vi "LeakageFenxi.vi"(7 "采样时间":string, 8 "Area_name":string, 9 "采样数据":string[][](array[string]), 10 "是否存在记录":bool=TRUE, 11 "3DData":cluster{"X":dbl[], "Y":dbl[], "Z":dbl[]}) -> ()   [LabVIEW 2014, in "cyy.lvlib" / "LeakageFenXi.lvlib"]
uses:
  LeakageFenXi.lvlib
  <vilib>/Math Plots/3D Math Plots/3D Contour/3D Contour XCtrl/3D Contour.xctl
  <vilib>/Math Plots/3D Math Plots/3D Surface/3D Surface XCtrl/3D Surface.xctl
  <vilib>/Math Plots/3D Math Plots/3D Mesh/3D Mesh XCtrl/3D Mesh.xctl
  <vilib>/imath/engines/lvmath2/RunTimeEngine/Managers/WorkSpace/UID Generator.vi
  <vilib>/imath/engines/lvmath2/RunTimeEngine/RunTimeType/NIMS_RunTimeType_From StrictType (excl LVString).vi
  <instcachedir>/0/NIMS_RunTimeType_From StrictType (excl LVString)_15A5391EEA9C4AACB9955AC755B83D29.lvgen/NIMS_RunTimeType_From StrictType (excl LVString)_15A5391EEA9C4AACB9955AC755B83D29_000.vi
  <vilib>/imath/engines/lvmath2/RunTimeEngine/LocalVariableDefStatement/MC_LocalVariableDefStatement_Display.vi
  <vilib>/imath/engines/lvmath2/RunTimeEngine/BuiltInFunctions/max/1 input/NIMS_max(RV).vi
  <instcachedir>/0/NIMS_max(RV)_237633DB1D604D5BA7001287DF3C7957.lvgen/NIMS_max(RV)_237633DB1D604D5BA7001287DF3C7957_000.vi
  <vilib>/imath/engines/lvmath2/RunTimeEngine/BuiltInFunctions/min/1 input/NIMS_min(RV).vi
  <instcachedir>/0/NIMS_min(RV)_EE2DD3E2888846108C5160A664B67832.lvgen/NIMS_min(RV)_EE2DD3E2888846108C5160A664B67832_000.vi
  <vilib>/imath/engines/lvmath2/RunTimeEngine/BuiltInFunctions/linramp/NIMS_linramp.vi
  <vilib>/imath/engines/lvmath2/RunTimeEngine/BuiltInFunctions/meshgrid2d/NIMS_meshgrid2d(V,V).vi
  <instcachedir>/0/NIMS_meshgrid2d(V,V)_3733343E1C554A708015CFB0432C6A59.lvgen/NIMS_meshgrid2d(V,V)_3733343E1C554A708015CFB0432C6A59_000.vi
  <vilib>/imath/engines/lvmath2/RunTimeEngine/BuiltInFunctions/intrp2d_uneven/NIMS_[1o]_intrp2d_uneven.vi
  <vilib>/imath/engines/lvmath2/RunTimeEngine/ErrorHandling/NIMS_Error From Error Code.vi
  <vilib>/imath/engines/lvmath2/RunTimeEngine/VariableToken/NIMS_VariableToken_CondDefined.vi
  <instcachedir>/0/NIMS_VariableToken_CondDefined_EE8DD211A89249938CE6537267F5C9B3.lvgen/NIMS_VariableToken_CondDefined_EE8DD211A89249938CE6537267F5C9B3_001.vi
  <vilib>/imathl/engines/lvmath/Functions/Error Handling/Create Error.vi
  <vilib>/imath/engines/lvmath/Functions/Error Handling/MergeErrorsWrapper.vi
  <vilib>/imath/engines/lvmath2/RunTimeEngine/Managers/SymbolTable/Clear UID.vi
  <vilib>/imath/engines/lvmath2/RunTimeEngine/NodeEndStatement/NIMS_NodeEndStatement_Output.vi
  <instcachedir>/0/NIMS_NodeEndStatement_Output_53EC0D466D134D7ABD903AC30B43404B.lvgen/NIMS_NodeEndStatement_Output_53EC0D466D134D7ABD903AC30B43404B_012.vi
  <instcachedir>/0/NIMS_NodeEndStatement_Output_53EC0D466D134D7ABD903AC30B43404B.lvgen/NIMS_NodeEndStatement_Output_53EC0D466D134D7ABD903AC30B43404B_002.vi
  <vilib>/imath/engines/lvmath2/RunTimeEngine/ErrorHandling/NIMS_Finalize Error.vi
  <vilib>/Utility/file.llb/Write To Spreadsheet File (string).vi
  <vilib>/imath/engines/lvmath2/RunTimeEngine/RangeToken/NIMS_Range_R2 - Integer.vi
  <instcachedir>/0/NIMS_Range_R2 - Integer_2D1304BAF97744E0A293025746CBADFC.lvgen/NIMS_Range_R2 - Integer_2D1304BAF97744E0A293025746CBADFC_000.vi
  <vilib>/imath/engines/lvmath2/RunTimeEngine/CommandStatement/MC_CommandStatement_break.vi
  <vilib>/imath/engines/lvmath2/RunTimeEngine/IndexRead/NIMS V(S).vi
  <instcachedir>/0/NIMS V(S)_0488751826AF41519A22953C041130DC.lvgen/NIMS V(S)_0488751826AF41519A22953C041130DC_000.vi
  <vilib>/imath/engines/lvmath2/RunTimeEngine/ArithmeticOperatorToken/NIMS_ArithmeticOperator_times.vi
  <instcachedir>/0/NIMS_ArithmeticOperator_times_2EFF5B13FCA4492A81D59089AD809F54.lvgen/NIMS_ArithmeticOperator_times_2EFF5B13FCA4492A81D59089AD809F54_007.vi
  <vilib>/imath/engines/lvmath2/RunTimeEngine/ArithmeticOperatorToken/NIMS_ArithmeticOperator_plus.vi
  <instcachedir>/0/NIMS_ArithmeticOperator_plus_48D6EAACA5D645B09F7EC9C016C2DEA8.lvgen/NIMS_ArithmeticOperator_plus_48D6EAACA5D645B09F7EC9C016C2DEA8_003.vi
  <vilib>/imath/engines/lvmath2/RunTimeEngine/ErrorHandling/NIMS_Create Error From Enums.vi
  <instcachedir>/0/NIMS_ArithmeticOperator_plus_48D6EAACA5D645B09F7EC9C016C2DEA8.lvgen/NIMS_ArithmeticOperator_plus_48D6EAACA5D645B09F7EC9C016C2DEA8_002.vi
  <vilib>/imath/engines/lvmath2/RunTimeEngine/BuiltInFunctions/abs/NIMS_abs(signed).vi
  <instcachedir>/0/NIMS_abs(signed)_C4FCB8E6058B49B797C7C8D53CA5F6EC.lvgen/NIMS_abs(signed)_C4FCB8E6058B49B797C7C8D53CA5F6EC_000.vi
  <instcachedir>/0/NIMS_ArithmeticOperator_times_2EFF5B13FCA4492A81D59089AD809F54.lvgen/NIMS_ArithmeticOperator_times_2EFF5B13FCA4492A81D59089AD809F54_001.vi
  <vilib>/imath/engines/lvmath2/RunTimeEngine/IndexReplace/NIMS M($,$)=M.vi
  <instcachedir>/0/NIMS M($,$)=M_01E89DEB123E4D8BA4D741A9F51B9E5E.lvgen/NIMS M($,$)=M_01E89DEB123E4D8BA4D741A9F51B9E5E_002.vi
  <vilib>/imath/engines/lvmath2/RunTimeEngine/IndexReplace/NIMS M(S,S)=S.vi
  <instcachedir>/0/NIMS M(S,S)=S_43446D47E75543269C90719353EB0EB0.lvgen/NIMS M(S,S)=S_43446D47E75543269C90719353EB0EB0_001.vi
  <vilib>/imath/engines/lvmath2/RunTimeEngine/IndexRead/NIMS M($,$).vi
  <instcachedir>/0/NIMS M($,$)_A19103A80C29478F88F4B4F0744DBFE6.lvgen/NIMS M($,$)_A19103A80C29478F88F4B4F0744DBFE6_000.vi
  <vilib>/imath/engines/lvmath2/RunTimeEngine/BuiltInFunctions/max/1 input/NIMS_max(CM).vi
  <instcachedir>/0/NIMS_max(CM)_07A280EFFE444116B5339E96F9201E32.lvgen/NIMS_max(CM)_07A280EFFE444116B5339E96F9201E32_000.vi
  <vilib>/imath/engines/lvmath2/RunTimeEngine/BuiltInFunctions/min/1 input/NIMS_min(CV).vi
  <instcachedir>/0/NIMS_min(CV)_813D140E220645C2A7BAD197162D0D3E.lvgen/NIMS_min(CV)_813D140E220645C2A7BAD197162D0D3E_000.vi
  <instcachedir>/0/NIMS V(S)_0488751826AF41519A22953C041130DC.lvgen/NIMS V(S)_0488751826AF41519A22953C041130DC_002.vi
  <instcachedir>/0/NIMS_NodeEndStatement_Output_53EC0D466D134D7ABD903AC30B43404B.lvgen/NIMS_NodeEndStatement_Output_53EC0D466D134D7ABD903AC30B43404B_005.vi
  <vilib>/Math Plots/3D Math Plots/3D Contour/3D Contour Datatype/Public/Plot Helper (Matrix).vi
  <vilib>/imath/engines/lvmath2/RunTimeEngine/BuiltInFunctions/max/1 input/NIMS_max(RM).vi
  <instcachedir>/0/NIMS_max(RM)_8387F852894F4122B05F4338BED9FDFF.lvgen/NIMS_max(RM)_8387F852894F4122B05F4338BED9FDFF_000.vi
  <vilib>/Math Plots/3D Math Plots/3D Surface/3D Surface Datatype/Public/Plot Helper (Matrix).vi
  <vilib>/Math Plots/3D Math Plots/3D Mesh/3D Mesh Datatype/Public/Plot Helper (Matrix).vi
  <vilib>/Math Plots/3D Math Plots/3D Contour/3D Contour Datatype/3D Contour Datatype.lvclass
  <vilib>/imath/engines/lvmath2/RunTimeEngine/Managers/SymbolTable/NIMS_WorkSpace.lvlib
  <vilib>/Math Plots/3D Math Plots/3D Surface/3D Surface Datatype/3D Surface Datatype.lvclass
  <vilib>/Math Plots/3D Math Plots/3D Mesh/3D Mesh Datatype/3D Mesh Datatype.lvclass
  CYY/cyy.lvlib
  DataBase/DataBase.lvlib
panel:
  in  "预警":bool
  in  "查看采样数据":bool
  out "当前采样分析信息":string
  out "最大索引":u32[](array[numeric])
  out "数字":dbl[](array[numeric]) format="%#.6g"
  out "数字 2":dbl[](array[numeric]) format="%#.6g"
  in  "退出":bool
  in  "分析":bool
  in  "预判":bool
  in  "预判方式":u16(ring) items=["linear", "cubic", "nearest"]
  in  "导出数据":bool
  in  "三维网格图":bool
  in  "三维曲面图":bool
  in  "三维等高线":bool
  out "预判点":string
  out "渗漏点":string
  in  "MMM":bool
  in  "选项卡控件":enum32{"三维曲面图", "三维等高线图", "三维网格图", "采样数据"}(tab)
  out "3D Surface":refnum<class "3D Plot Datatype.lvclass">[](xcontrol) caption="三维曲面"
  out "3D等高线":refnum<class "3D Plot Datatype.lvclass">[](xcontrol) caption="三维等高线"
  out "3D Mesh":refnum<class "3D Plot Datatype.lvclass">[](xcontrol) caption="三维网格"
  in  "采样数据":i32(listbox)
  out "导出数据位置":path
  out "Z索引":i32
  out "Y坐标":dbl
  out "X坐标":dbl
  out "Zmax":dbl
  out "绘图坐标Y":dbl
  out "绘图坐标X":dbl
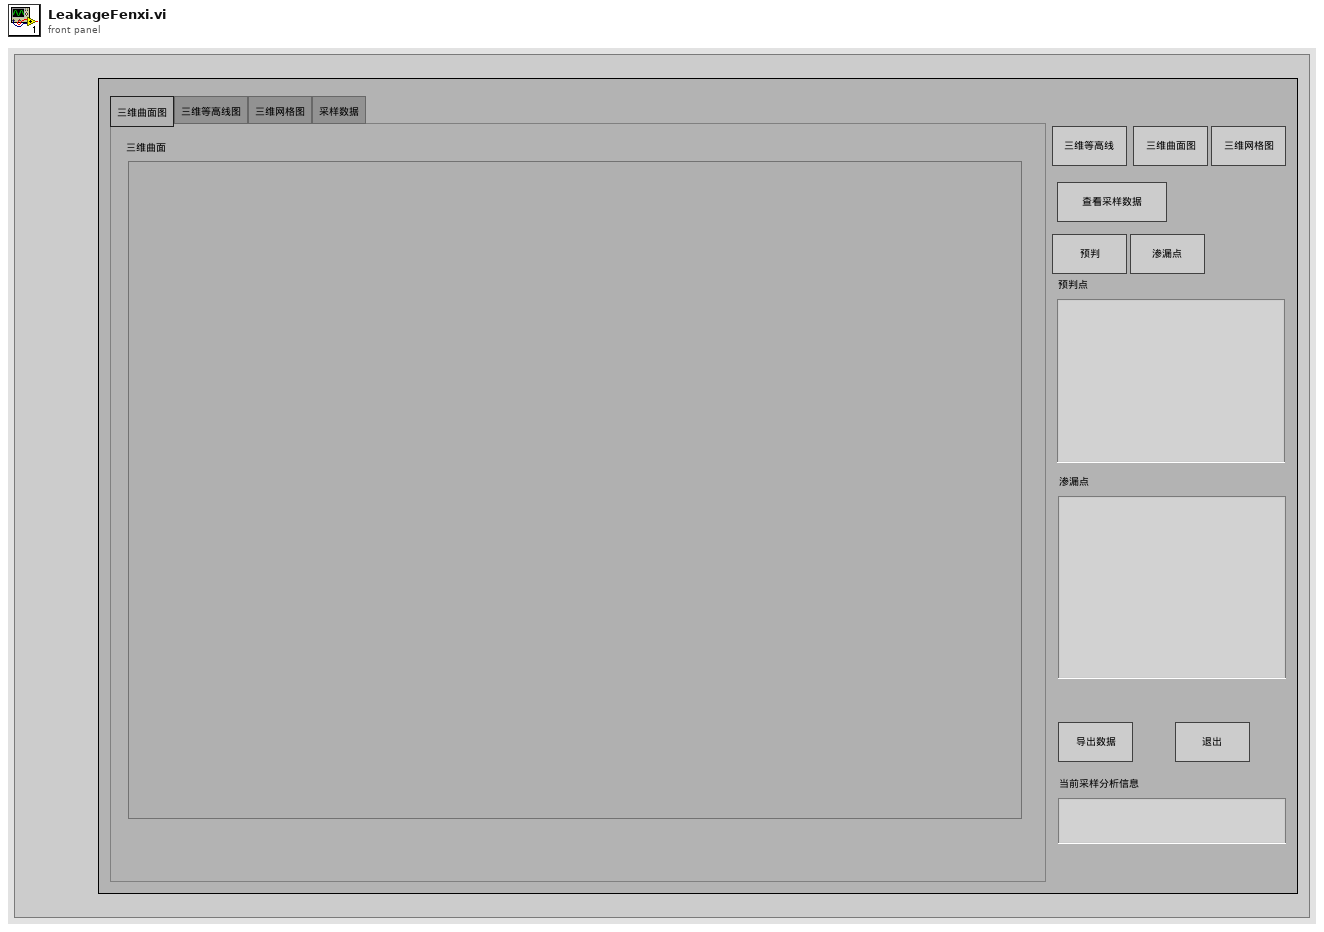
[diagram p1: front panel]
types:
  T1 = enum32{"invalid app kind", "Development System", "Run Time System", "Student Edition", "Embedded LabVIEW", "Evaluation", "Custom"}
  T2 = enum32{"Invalid", "Standard", "Closed", "Hidden", "Minimized", "Maximized"}
  T3 = cluster{"Core":cluster{"Current VI Reference":refnum<vi>, "Close Panel on Exit?":bool}, "Your Boolean data":bool, "Your string data":string, "3DData":cluster{"X":dbl[], "Y":dbl[], "Z":dbl[]}, "是否存在记录":bool, "采样数据":string[][], "SampleTime":string, "插值方式":i32, "Area_name":string, "坐标关系":cluster{"绘图坐标X":string, "绘图坐标Y":string, "实际坐标":string[]}, "是否进行预判":bool, "是否进行预警":bool}
  T4 = cluster{"绘图坐标X":string, "绘图坐标Y":string, "实际坐标":string[]}
  T5 = cluster{"Current VI Reference":refnum<vi>, "Close Panel on Exit?":bool}
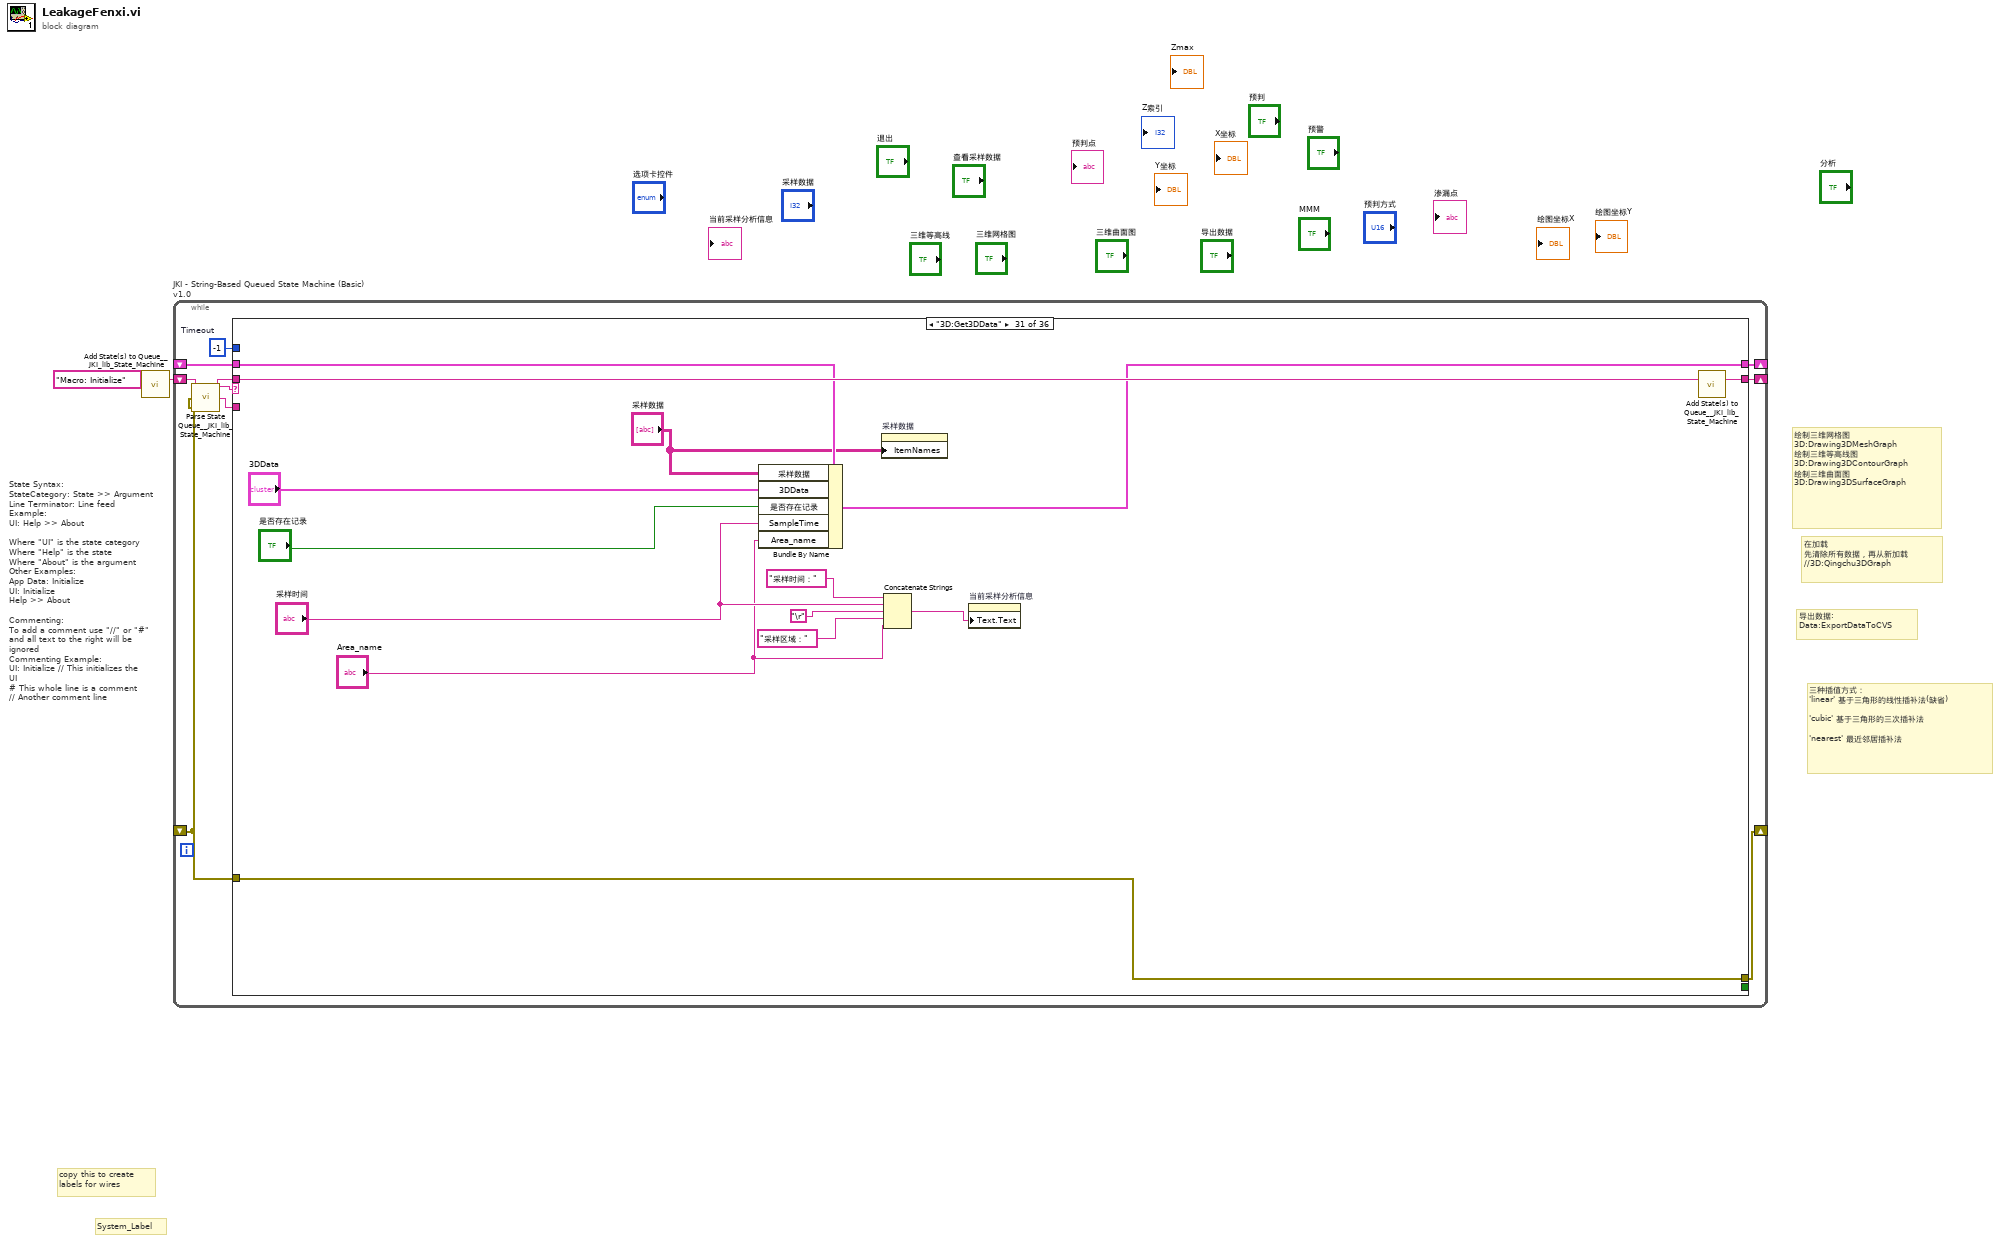
[diagram p0: block diagram]
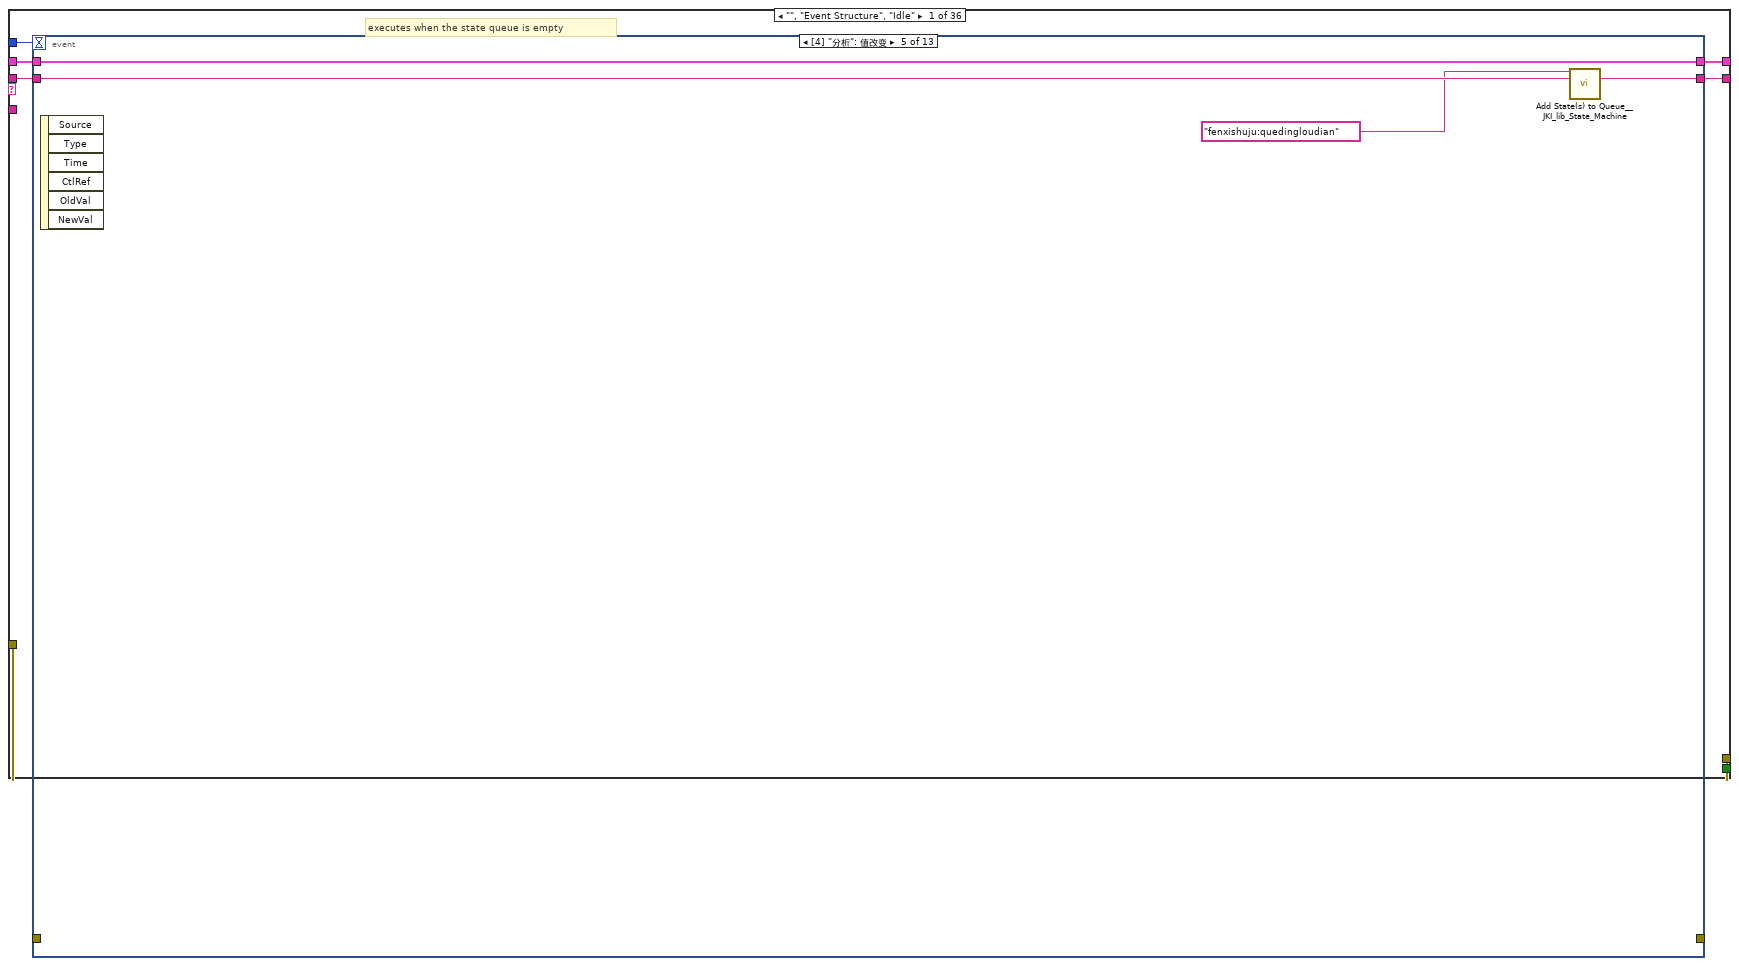
[diagram p2: hidden frame]
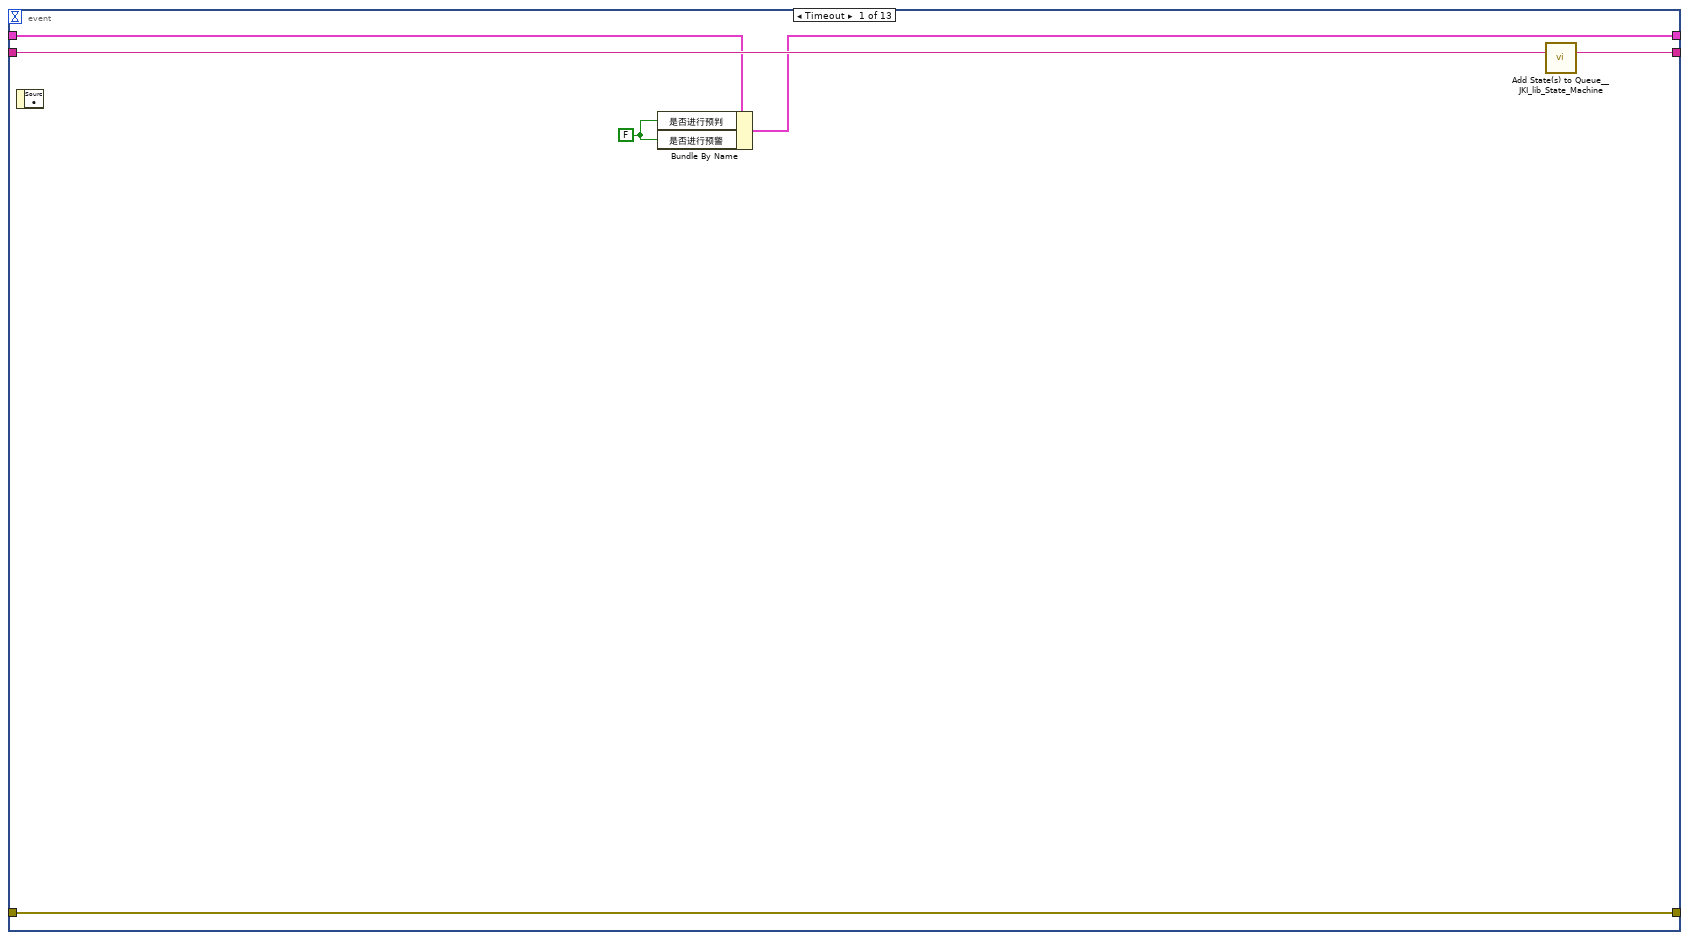
[diagram p3: hidden frame]
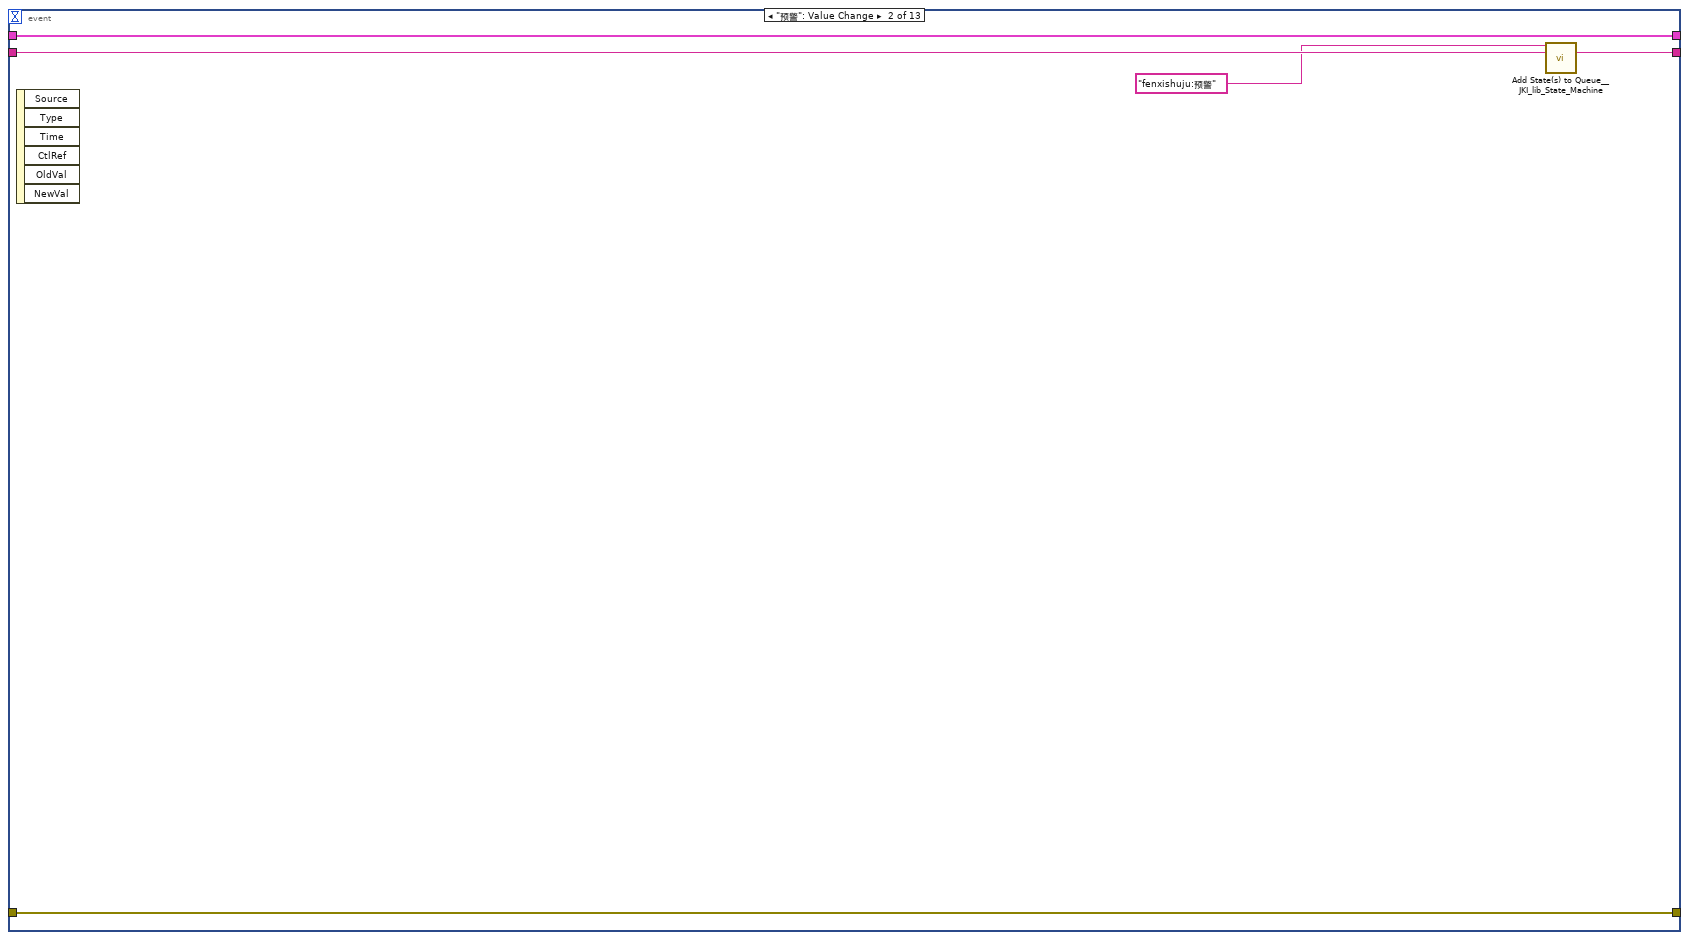
[diagram p4: hidden frame]
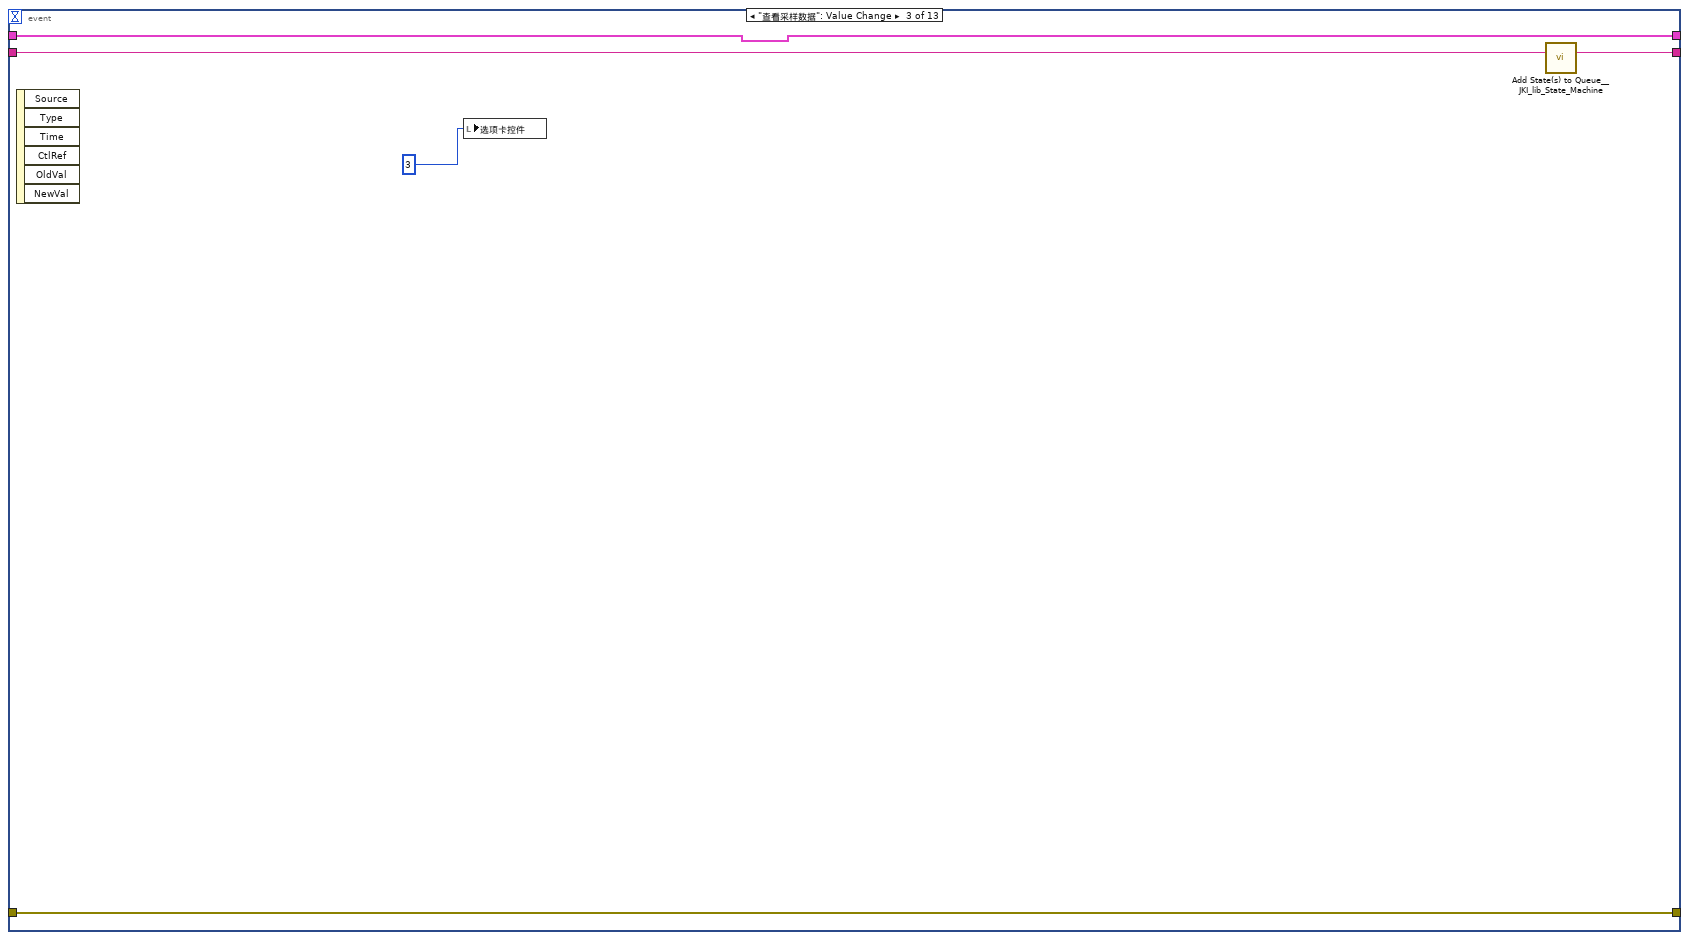
[diagram p5: hidden frame]
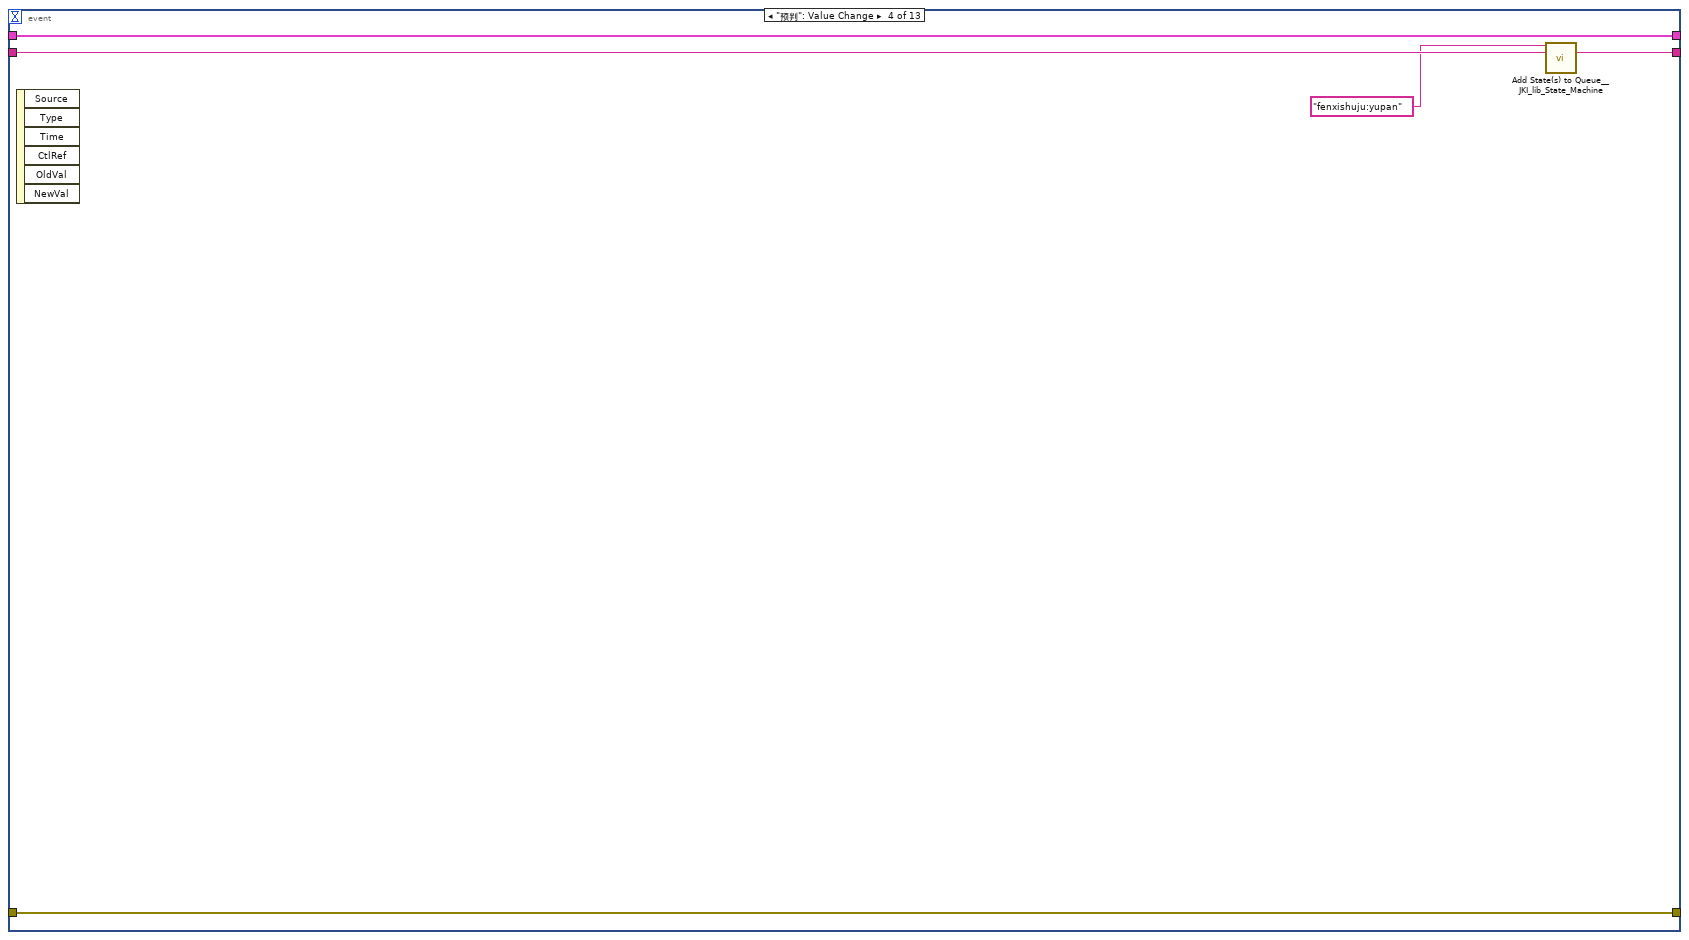
[diagram p6: hidden frame]
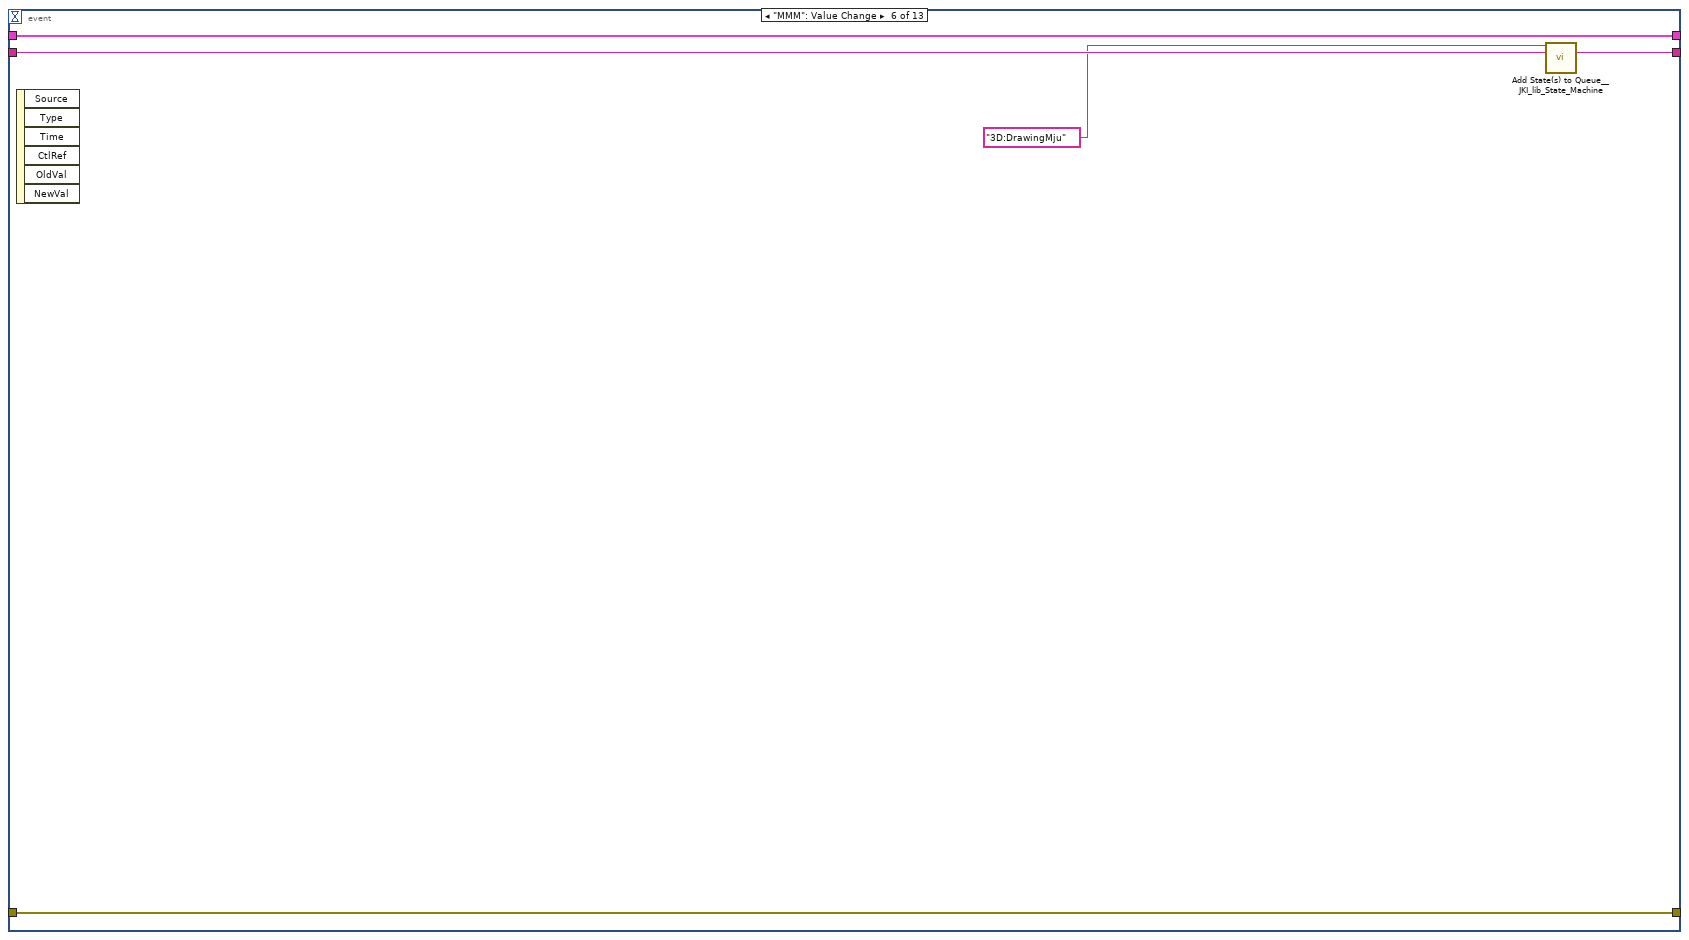
[diagram p7: hidden frame]
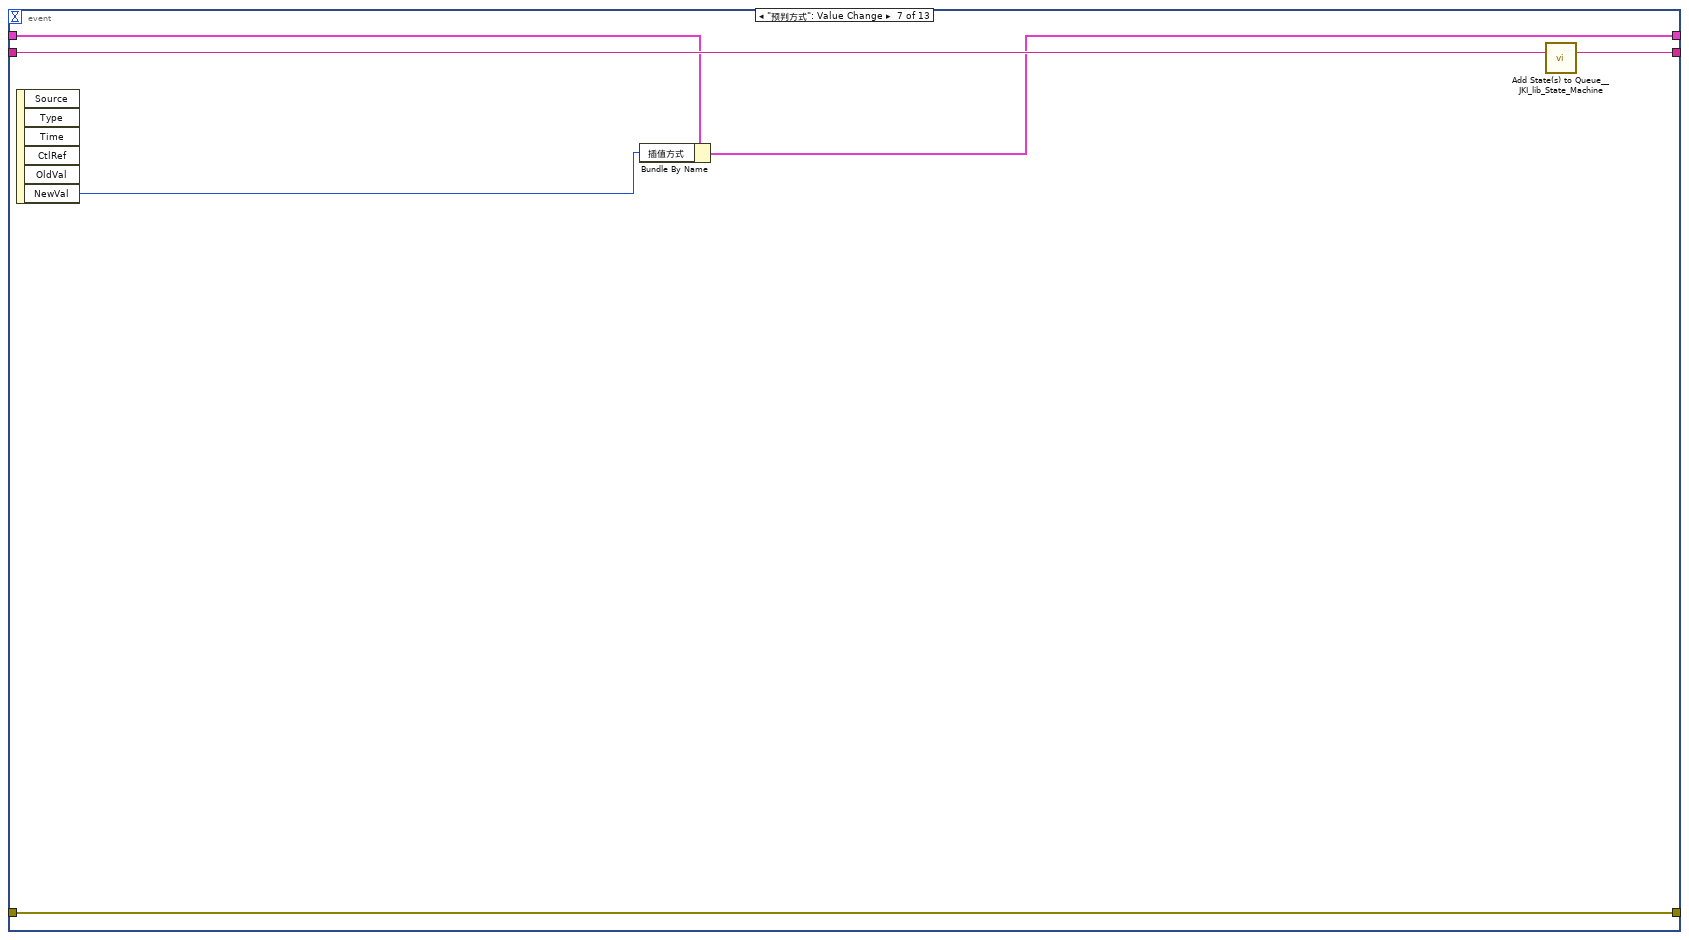
[diagram p8: hidden frame]
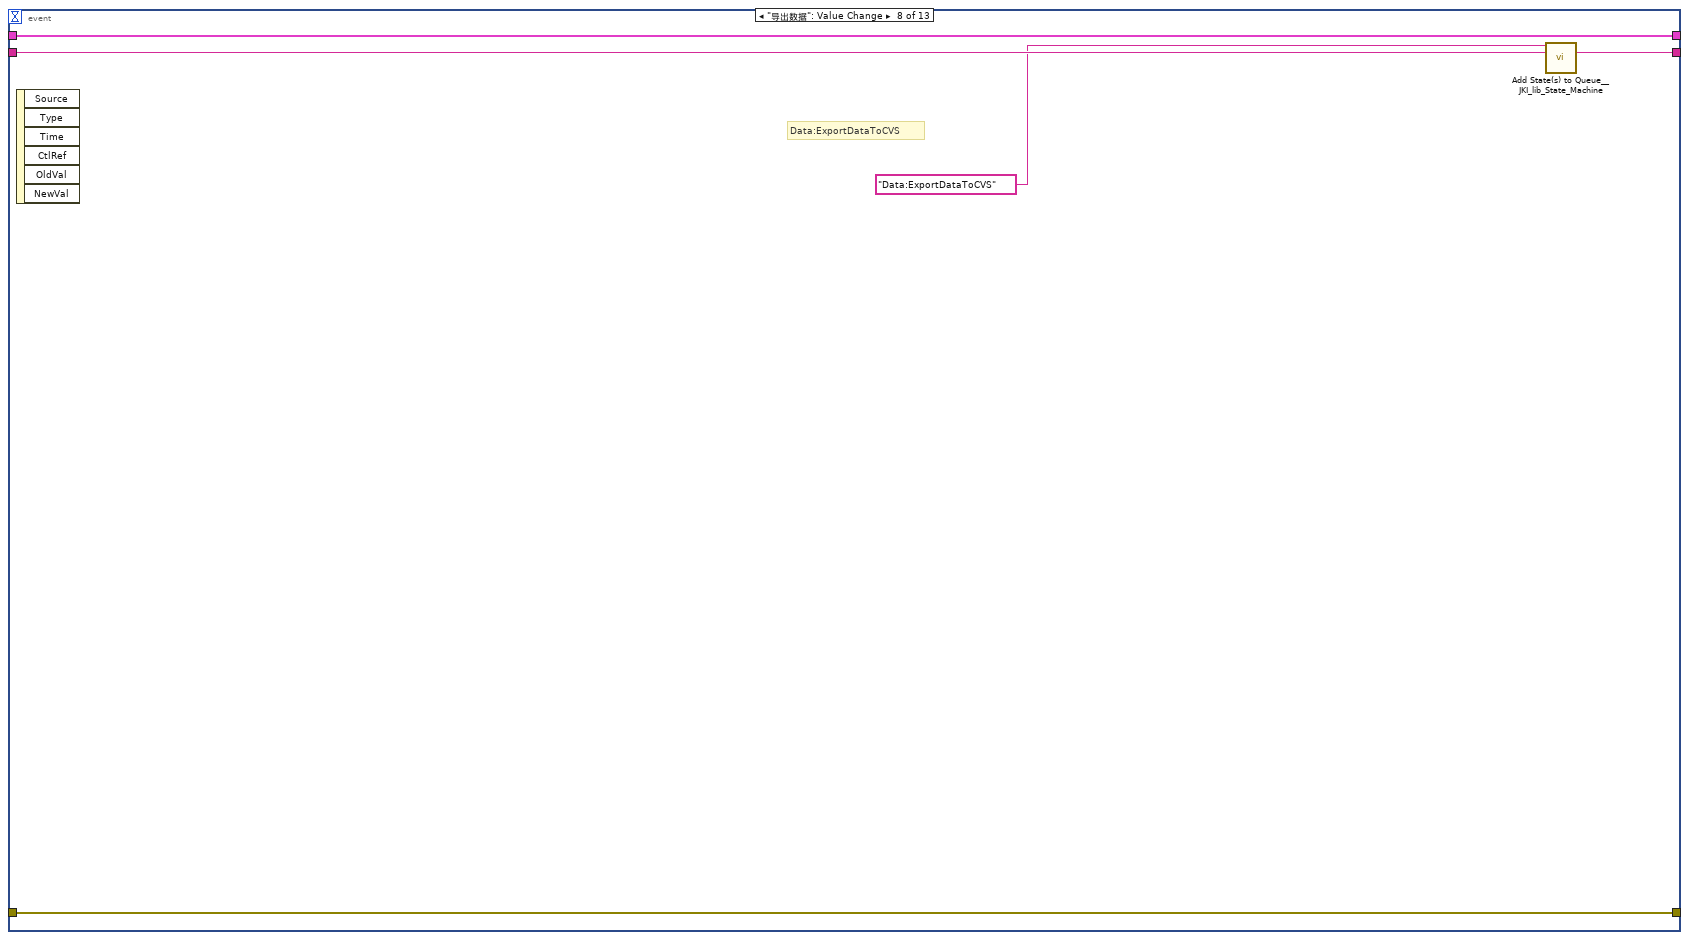
[diagram p9: hidden frame]
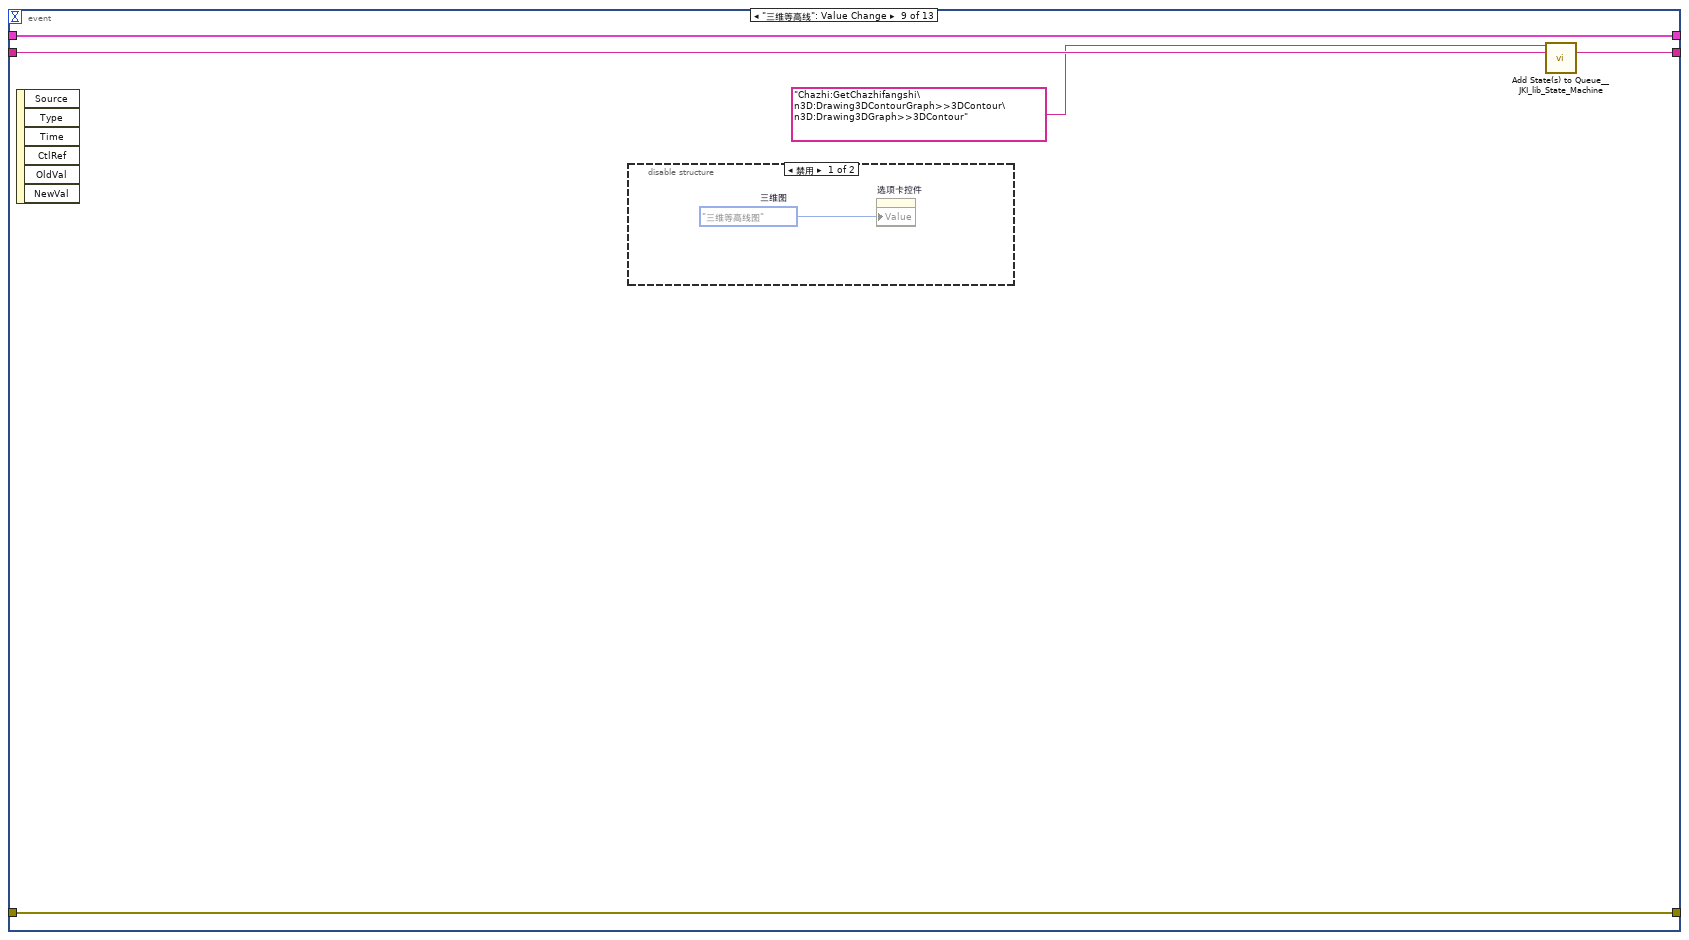
[diagram p10: hidden frame]
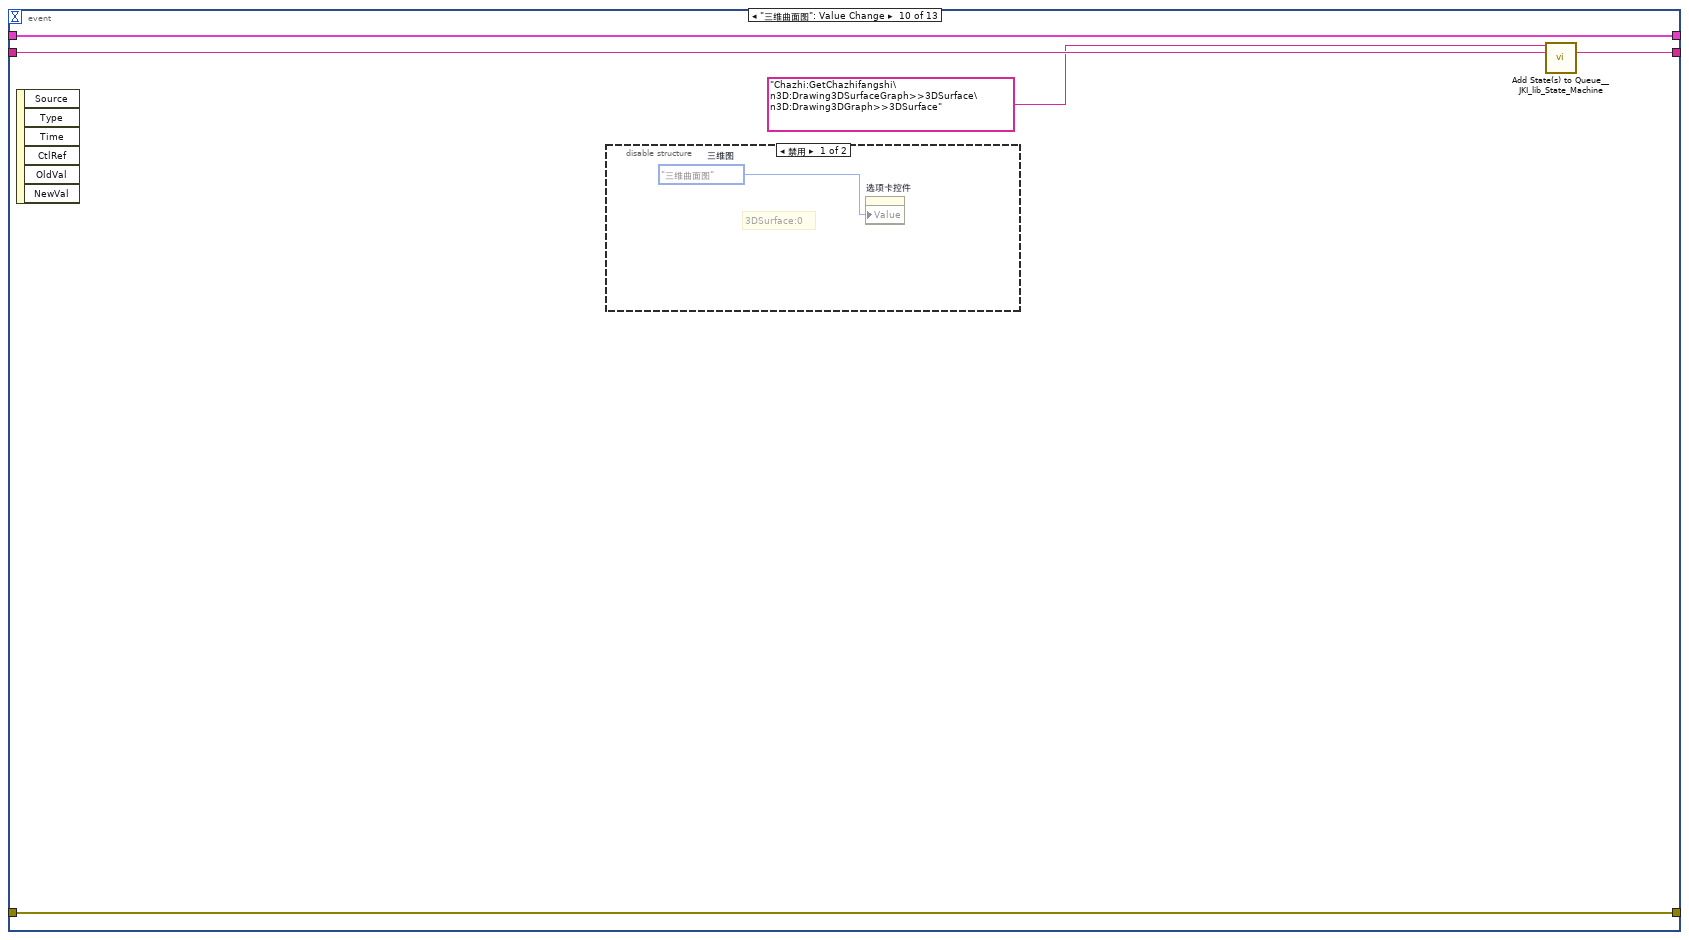
[diagram p12: hidden frame]
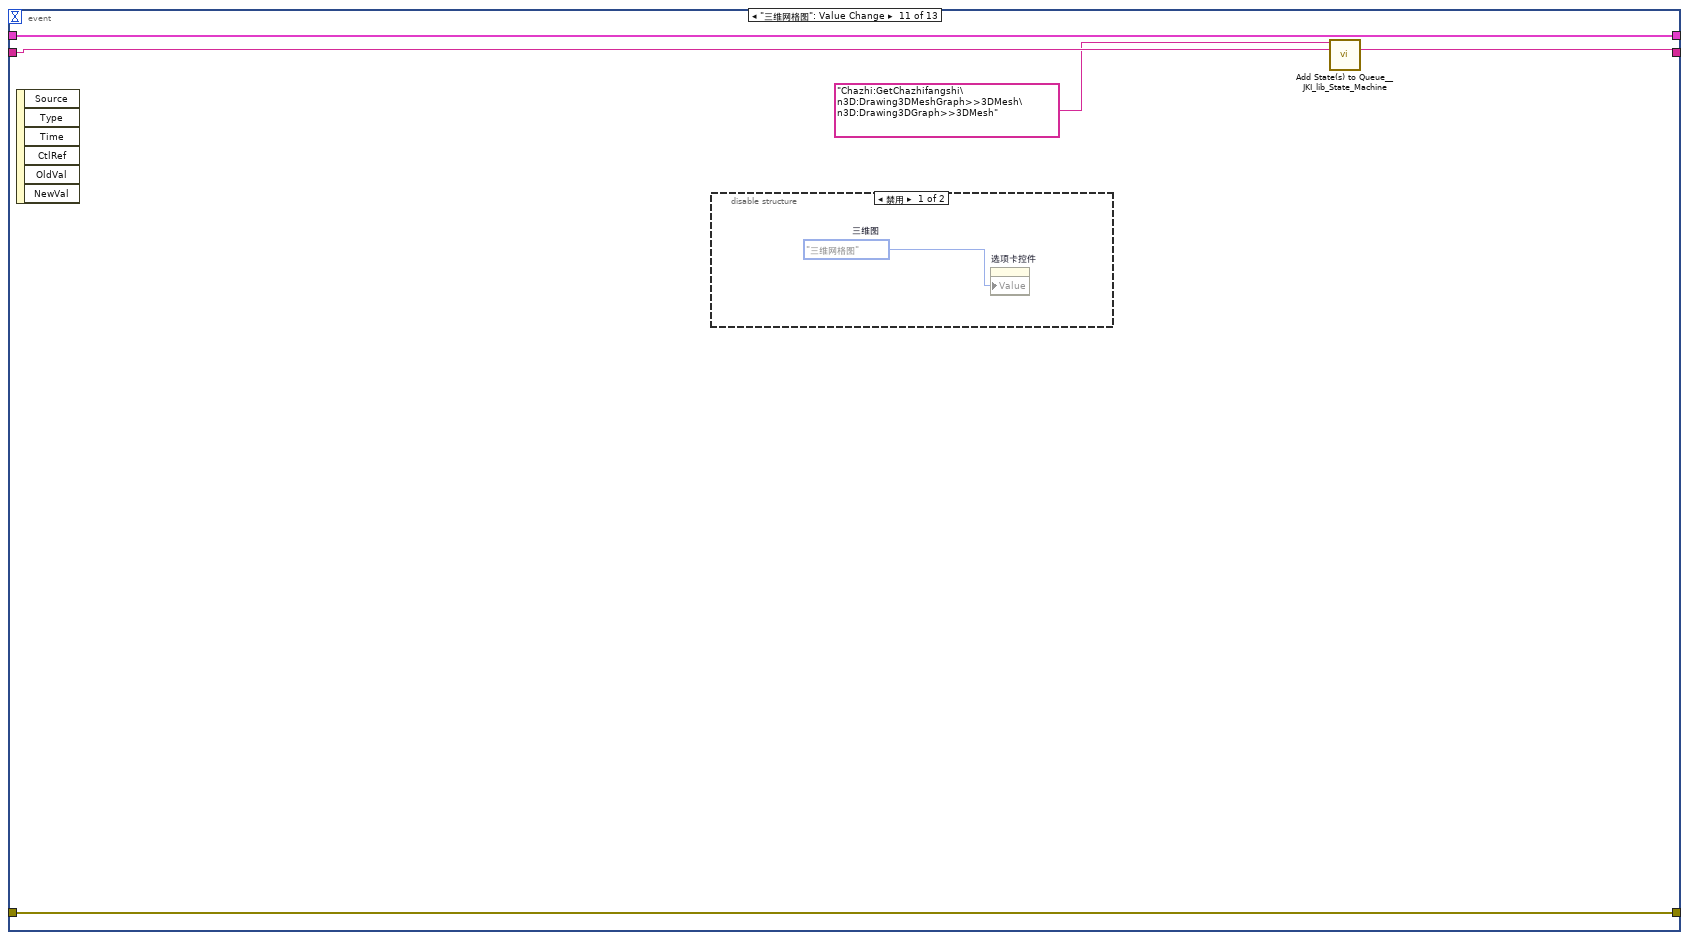
[diagram p14: hidden frame]
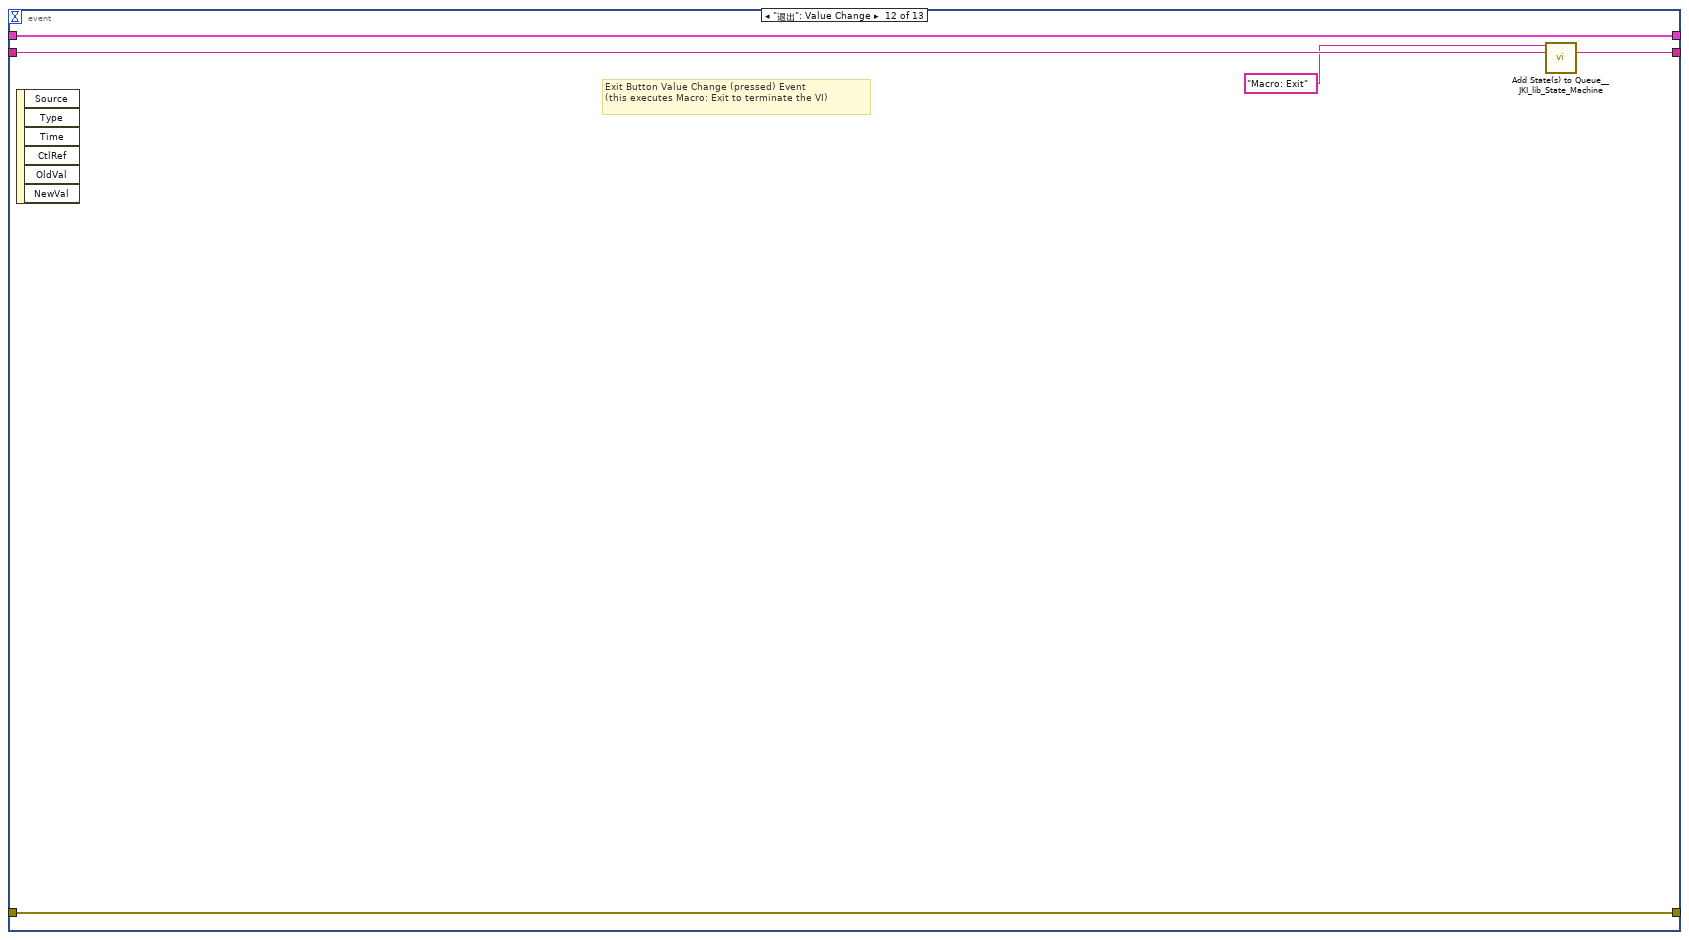
[diagram p16: hidden frame]
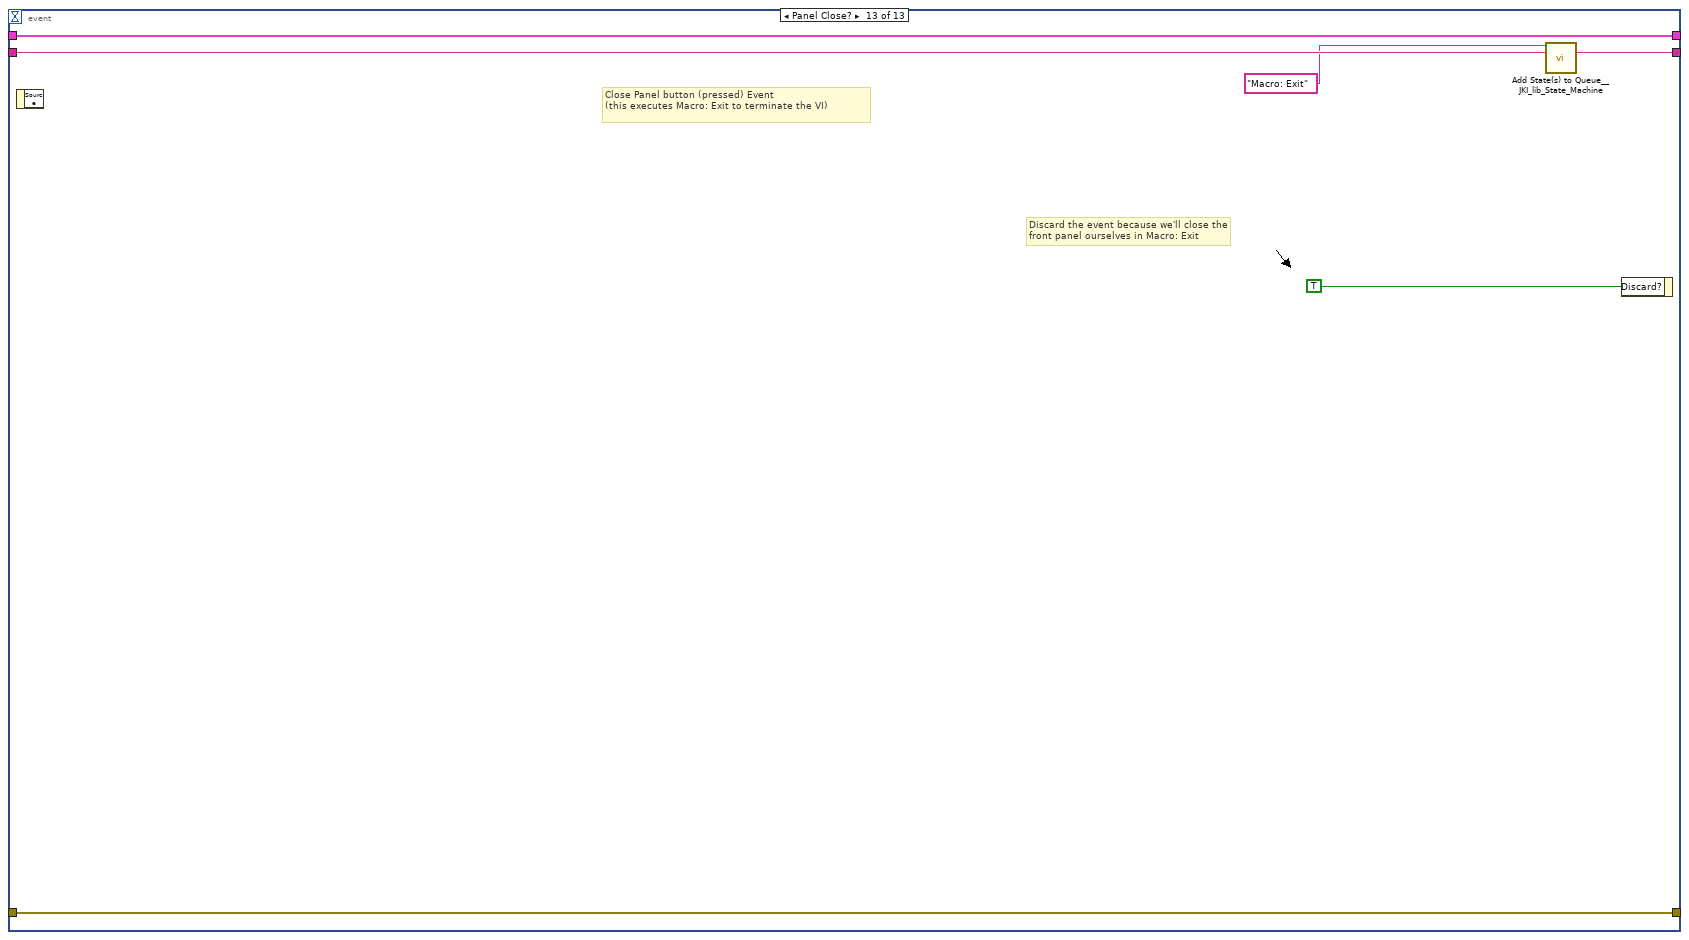
[diagram p17: hidden frame]
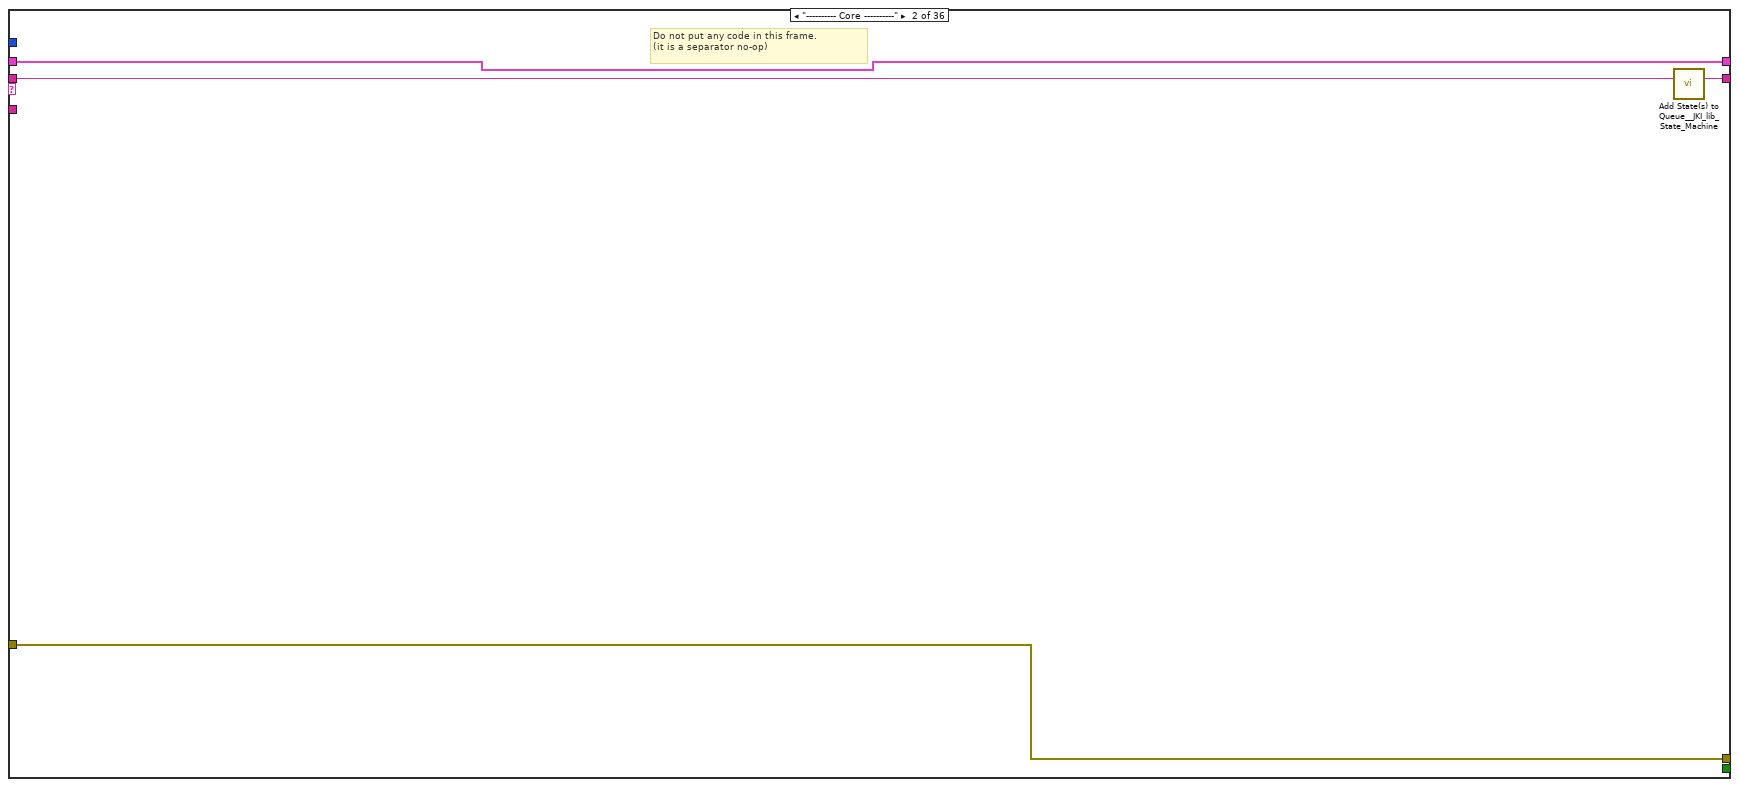
[diagram p18: hidden frame]
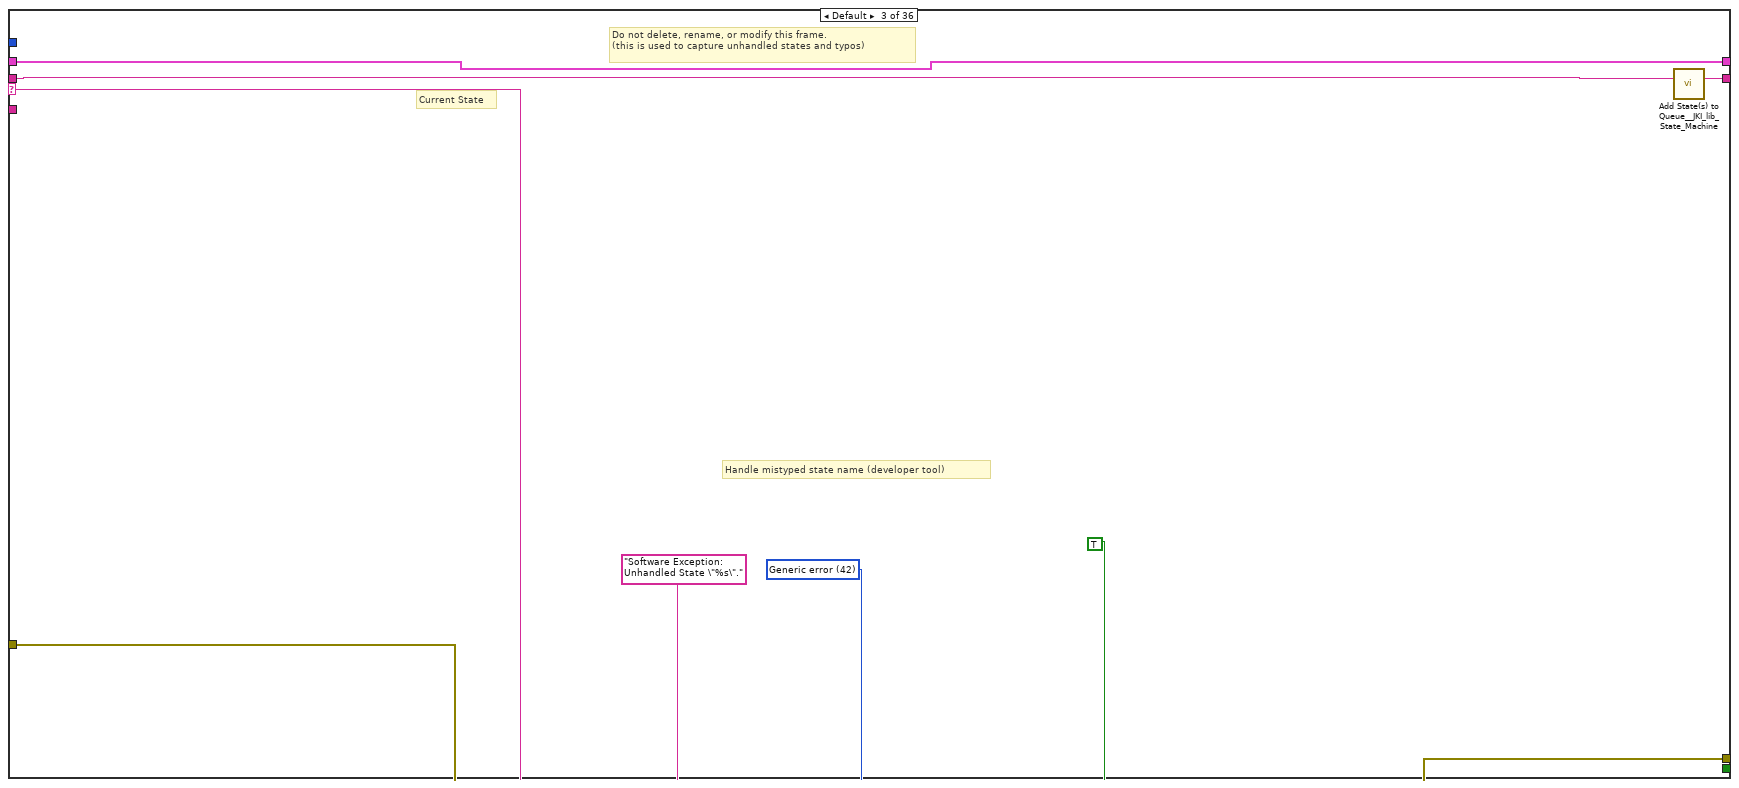
[diagram p19: hidden frame]
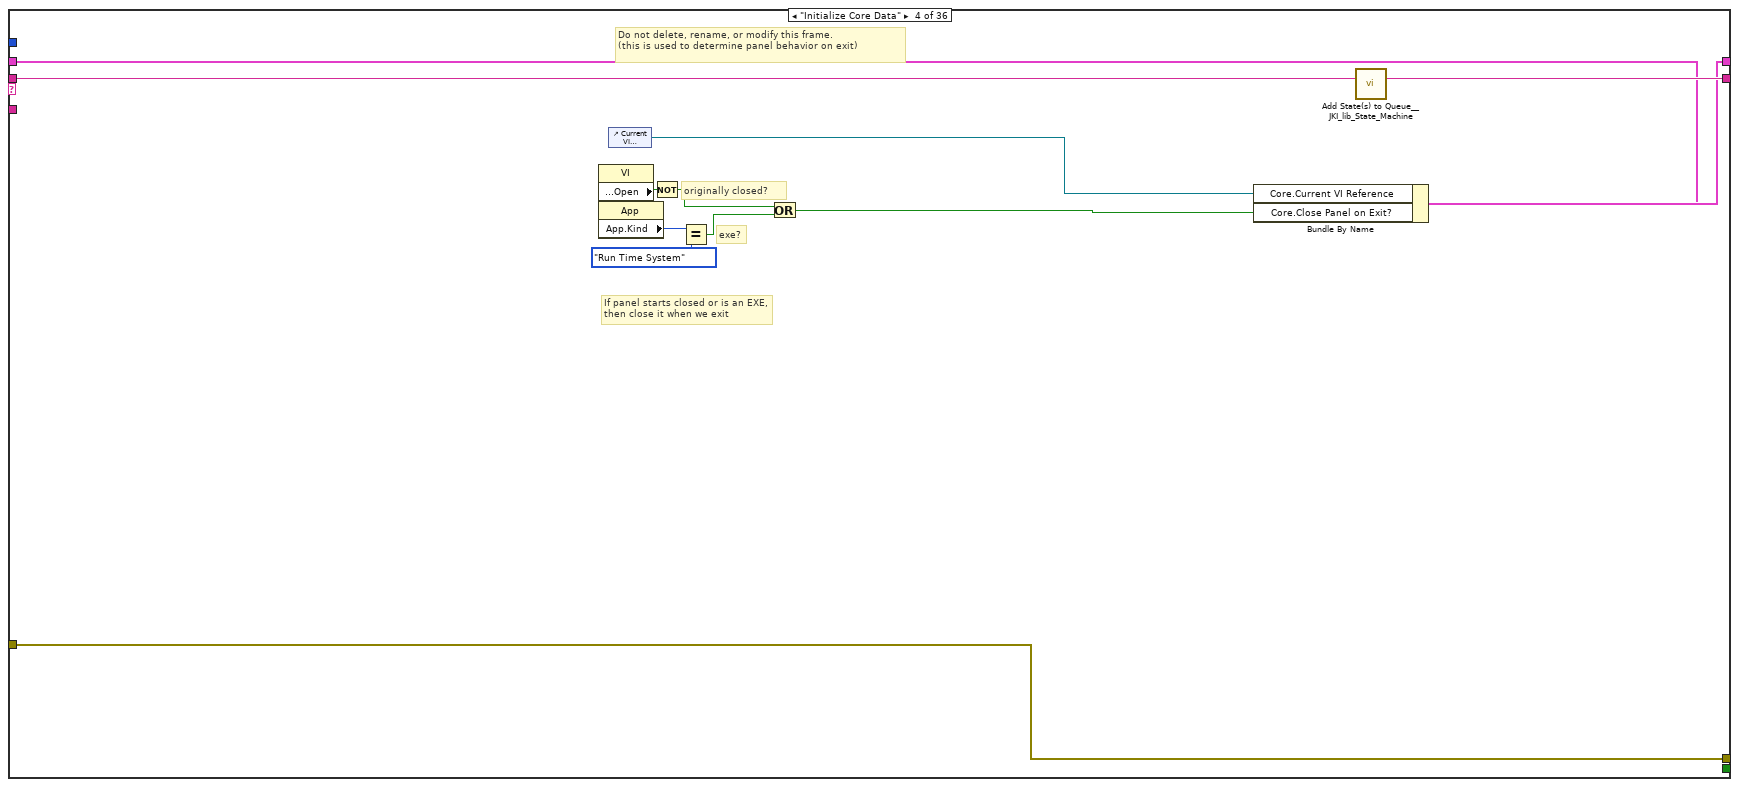
[diagram p20: hidden frame]
diagram:
  # "三种插值方式：\n'linear' 基于三角形的线性插补法(缺省)\n\n'cubic' 基于三角形的三次插补法\n\n'nearest' 最近邻居插补法"
  # "在加载\n先清除所有数据，再从新加载\n//3D:Qingchu3DGraph"
  # "导出数据:\nData:ExportDataToCVS"
  # "绘制三维网格图\n3D:Drawing3DMeshGraph\n绘制三维等高线图\n3D:Drawing3DContourGraph\n绘制三维曲面图\n3D:Drawing3DSurfaceGraph"
  # "State Syntax:\nStateCategory: State >> Argument\nLine Terminator: Line feed\nExample:\nUI: Help >> About\n\nWhere \"UI\" is the state category\nWhere \"Help\" is the state\nWhere \"About\" is the argument\nOther Examples:\nApp Data: Initialize\nUI: Initialize\nHelp >> About\n\nCommenting:\nTo add a comment use \"//\" or \"#\" and all text to the right will be ignored\nCommenting Example:\nUI: Initialize // This initializes the UI\n# This whole line is a comment\n// Another comment line"
  # "copy this to create labels for wires"
  # "System_Label"
  n1 = call <vilib>:"Add State(s) to Queue__JKI_lib_State_Machine.vi"("State(s) in (\"\")"="Macro: Initialize") -> ("States Out"=w2:string)  [unwired: 14 in]
  n2 = while "JKI - String-Based Queued State Machine (Basic) v1.0" {
    shift-right: [w6] -> _
    shift-left: _ -> [w5]
    shift-right: [w9] -> _
    shift-left: _ -> [w3]
    shift-right: [w8] -> _
    shift-left: w2 -> [w10]
    stop <- w7 stop-if-true
    w4 = -1  # Timeout
    n3 = call <vilib>:"Parse State Queue__JKI_lib_State_Machine.vi"("State Queue"=w10, "Error In (no error)"=w3) -> ("Remaining States"=w12:string, "Current State"=w13:string, "Arguments"=w11:string)  [unwired: 11 in]
    n4 = case shown="\"3D:Get3DData\"" w13 {
      selector: w13 -> [_ _ w96 _ _ _ _ _ _ _ _ _ _ _ _ _ _ _ _ _ _ _ _ _ _ _ _ _ _ _ _ _ _ _ _ _]
      tunnel: w12 -> [w20 w95 w100 w118 w124 w129 w133 w149 w155 w159 w165 w171 w182 w208 w215 w228 w232 w236 w240 w244 w259 w305 w642 w646 w652 w656 w662 w697 w704 w2135 w2149 w2160 w2453 w2773 w3095 w3385]
      tunnel: w11 -> [_ _ _ _ _ _ _ _ _ _ _ w166 w176 _ _ _ _ _ _ _ _ _ _ _ _ _ _ _ _ _ _ _ _ _ _ w3381]
      tunnel: w5 -> [w18 w92 w98 w109 w121 w127 w130 _ w150 w156 w163 w169 w178 w205 w210 w225 w229 w233 w237 w241 w256 w297 w624 w643 w648 w653 w659 w694 w701 w2132 w2145 w2157 w2450 w2770 w3092 w3382]
      tunnel: [w17 w93 w102 w115 errorcluster {"status"=FALSE, "code"=0, "source"=""} ("error out") w126 w131 w146 w151 w157 w162 w167 w179 w206 w213 w226 w230 w234 w238 w242 w257 w303 w640 w644 w650 w654 w660 w695 w702 w2133 w2147 w2158 w2451 w2771 w3093 w3383] -> w9
      tunnel: w3 -> [w16 w93 w101 w115 w120 w126 w131 w146 w152 w157 w162 w168 w180 w206 w213 w226 w230 w234 w238 w242 w257 w303 w640 w644 w650 w654 w660 w695 w702 w2133 w2147 w2158 w2451 w2771 w3093 w3383]
      tunnel: [w19 w94 w99 w117 w123 w128 w132 w148 w154 w158 w164 w170 w181 w207 w214 w227 w231 w235 w239 w243 w258 w304 w641 w645 w651 w655 w661 w696 w703 w2134 w2148 w2159 w2452 w2772 w3094 w3384] -> w8
      tunnel: [_ _ _ _ _ TRUE _ _ _ _ _ _ _ _ _ _ _ _ _ _ _ _ _ _ _ _ _ _ _ _ _ _ _ _ _ _] -> w7
      tunnel: [w15 w92 w98 w116 w121 w127 w130 w147 w150 w156 w163 w169 w178 w205 w209 w225 w229 w233 w237 w241 w255 w296 w623 w643 w647 w653 w659 w694 w701 w2132 w2144 w2157 w2450 w2770 w3092 w3382] -> w6
      tunnel: w4 -> [w14 _ _ _ _ _ _ _ _ _ _ _ _ _ _ _ _ _ _ _ _ _ _ _ _ _ _ _ _ _ _ _ _ _ _ _]
      frame "", "Event Structure", "Idle" {
        # "executes when the state queue is empty"
        n5 = event shown="[4] \"分析\": 值改变" {
          selector: _ -> [_ _ _ _ _ _ _ _ _ _ _ _ _]
          dyn-events: _ -> [_ _ _ _ _ _ _ _ _ _ _ _ _]
          timeout: w14 -> [_ _ _ _ _ _ _ _ _ _ _ _ _]
          tunnel: w20 -> [w26 w31 w36 w41 w46 w51 w57 w62 w67 w73 w79 w85 w91]
          tunnel: [w25 w30 w35 w40 w45 w50 w56 w61 w66 w72 w78 w84 w90] -> w19
          tunnel: w18 -> [w23 w28 w33 w38 w43 w48 w53 w59 w64 w70 w77 w82 w88]
          tunnel: [w24 w29 w34 w39 w44 w49 w55 w60 w65 w71 w76 w83 w89] -> w17
          tunnel: w16 -> [w24 w29 w34 w39 w44 w49 w55 w60 w65 w71 w76 w83 w89]
          tunnel: [w22 w28 w33 w38 w43 w48 w52 w59 w64 w70 w77 w82 w88] -> w15
          event Timeout {
            w21 = FALSE
            n6 = event-data() -> ()  [unwired: 1 in, 1 out]
            n7 = Bundle By Name(cluster=w23, "是否进行预判"=w21, "是否进行预警"=w21) -> (w22:T3)
            n8 = call <vilib>:"Add State(s) to Queue__JKI_lib_State_Machine.vi"("State(s) in (\"\")"=w26) -> ("States Out"=w25:string)  [unwired: 14 in]
          }
          event "预警": Value Change {
            n9 = event-data() -> ()  [unwired: 1 in, 6 out]
            n10 = call <vilib>:"Add State(s) to Queue__JKI_lib_State_Machine.vi"("State(s) in Front (\"\")"="fenxishuju:预警", "State(s) in (\"\")"=w31) -> ("States Out"=w30:string)  [unwired: 13 in]
          }
          event "查看采样数据": Value Change {
            n11 = event-data() -> ()  [unwired: 1 in, 6 out]
            n12 = local write "选项卡控件"(3) -> ()
            n13 = call <vilib>:"Add State(s) to Queue__JKI_lib_State_Machine.vi"("State(s) in (\"\")"=w36) -> ("States Out"=w35:string)  [unwired: 14 in]
          }
          event "预判": Value Change {
            n14 = event-data() -> ()  [unwired: 1 in, 6 out]
            n15 = call <vilib>:"Add State(s) to Queue__JKI_lib_State_Machine.vi"("State(s) in Front (\"\")"="fenxishuju:yupan", "State(s) in (\"\")"=w41) -> ("States Out"=w40:string)  [unwired: 13 in]
          }
          event "分析": Value Change {
            n16 = event-data() -> ()  [unwired: 1 in, 6 out]
            n17 = call <vilib>:"Add State(s) to Queue__JKI_lib_State_Machine.vi"("State(s) in Front (\"\")"="fenxishuju:quedingloudian", "State(s) in (\"\")"=w46) -> ("States Out"=w45:string)  [unwired: 13 in]
          }
          event "MMM": Value Change {
            n18 = event-data() -> ()  [unwired: 1 in, 6 out]
            n19 = call <vilib>:"Add State(s) to Queue__JKI_lib_State_Machine.vi"("State(s) in Front (\"\")"="3D:DrawingMju", "State(s) in (\"\")"=w51) -> ("States Out"=w50:string)  [unwired: 13 in]
          }
          event "预判方式": Value Change {
            n20 = event-data() -> ("NewVal"=w54:u16)  [unwired: 1 in, 5 out]
            n21 = Bundle By Name(cluster=w53, "插值方式"=w54) -> (w52:T3)
            n22 = call <vilib>:"Add State(s) to Queue__JKI_lib_State_Machine.vi"("State(s) in (\"\")"=w57) -> ("States Out"=w56:string)  [unwired: 14 in]
          }
          event "导出数据": Value Change {
            # "Data:ExportDataToCVS"
            n23 = event-data() -> ()  [unwired: 1 in, 6 out]
            n24 = call <vilib>:"Add State(s) to Queue__JKI_lib_State_Machine.vi"("State(s) in Front (\"\")"="Data:ExportDataToCVS", "State(s) in (\"\")"=w62) -> ("States Out"=w61:string)  [unwired: 13 in]
          }
          event "三维等高线": Value Change {
            n25 = event-data() -> ()  [unwired: 1 in, 6 out]
            n26 = disable-structure shown="禁用" {
              frame Disabled {
                w68 = enum32{"三维曲面图", "三维等高线图", "三维网格图"}."三维等高线图"  # 三维图
                n27 = property on="选项卡控件" class="TabCtl (严格)"("Value"=w68) -> ()  [unwired: 2 in, 2 out]
              }
              frame Enabled {
              }
            }
            n28 = call <vilib>:"Add State(s) to Queue__JKI_lib_State_Machine.vi"("State(s) in Front (\"\")"="Chazhi:GetChazhifangshi\n3D:Drawing3DContourGraph>>3DContour\n3D:Drawing3DGraph>>3DContour", "State(s) in (\"\")"=w67) -> ("States Out"=w66:string)  [unwired: 13 in]
          }
          event "三维曲面图": Value Change {
            n29 = event-data() -> ()  [unwired: 1 in, 6 out]
            n30 = disable-structure shown="禁用" {
              frame Disabled {
                w74 = enum32{"三维曲面图", "三维等高线图", "三维网格图"}."三维曲面图"  # 三维图
                # "3DSurface:0"
                n31 = property on="选项卡控件" class="TabCtl (严格)"("Value"=w74) -> ()  [unwired: 2 in, 2 out]
              }
              frame Enabled {
              }
            }
            n32 = call <vilib>:"Add State(s) to Queue__JKI_lib_State_Machine.vi"("State(s) in Front (\"\")"="Chazhi:GetChazhifangshi\n3D:Drawing3DSurfaceGraph>>3DSurface\n3D:Drawing3DGraph>>3DSurface", "State(s) in (\"\")"=w73) -> ("States Out"=w72:string)  [unwired: 13 in]
          }
          event "三维网格图": Value Change {
            n33 = event-data() -> ()  [unwired: 1 in, 6 out]
            n34 = disable-structure shown="禁用" {
              frame Disabled {
                w80 = enum32{"三维曲面图", "三维等高线图", "三维网格图"}."三维网格图"  # 三维图
                n35 = property on="选项卡控件" class="TabCtl (严格)"("Value"=w80) -> ()  [unwired: 2 in, 2 out]
              }
              frame Enabled {
              }
            }
            n36 = call <vilib>:"Add State(s) to Queue__JKI_lib_State_Machine.vi"("State(s) in Front (\"\")"="Chazhi:GetChazhifangshi\n3D:Drawing3DMeshGraph>>3DMesh\n3D:Drawing3DGraph>>3DMesh", "State(s) in (\"\")"=w79) -> ("States Out"=w78:string)  [unwired: 13 in]
          }
          event "退出": Value Change {
            # "Exit Button Value Change (pressed) Event\n(this executes Macro: Exit to terminate the VI)"
            n37 = event-data() -> ()  [unwired: 1 in, 6 out]
            n38 = call <vilib>:"Add State(s) to Queue__JKI_lib_State_Machine.vi"("State(s) in Front (\"\")"="Macro: Exit", "State(s) in (\"\")"=w85) -> ("States Out"=w84:string)  [unwired: 13 in]
          }
          event Panel Close? {
            # "Discard the event because we'll close the front panel ourselves in Macro: Exit"
            # "Close Panel button (pressed) Event\n(this executes Macro: Exit to terminate the VI)"
            n39 = event-data() -> ()  [unwired: 1 in, 1 out]
            n40 = call <vilib>:"Add State(s) to Queue__JKI_lib_State_Machine.vi"("State(s) in Front (\"\")"="Macro: Exit", "State(s) in (\"\")"=w91) -> ("States Out"=w90:string)  [unwired: 13 in]
            n41 = event-data("Discard?"=TRUE) -> ()  [unwired: 1 in, 1 out]
          }
        }
      }
      frame "---------- Core ----------" {
        # "Do not put any code in this frame.\n(it is a separator no-op)"
        n42 = call <vilib>:"Add State(s) to Queue__JKI_lib_State_Machine.vi"("State(s) in (\"\")"=w95) -> ("States Out"=w94:string)  [unwired: 14 in]
      }
      frame Default {
        w105 = 42 items=["No error", "Argument error", "Memory is full", "Out of zone", "End of file", "File already open", "Generic file I/O error", "File not found", "File permission error", "Disk is full", "Duplicate path", "Too many files open", "System feature not enabled", "Resource file not found", "Cannot add resource", "Resource not found", "Image not found", "Image memory error", "Pen does not exist", "Config type invalid", "Config token not found", "Config parse error", "Config memory error", "Bad external code format", "Bad external code offset", "External code not present", "Null window", "Destroy window error", "Null menu", "Print aborted", "Bad print record", "Print driver error", "Windows error during printing", "Memory error during printing", "Print dialog error", "Generic print error", "Invalid device refnum", "Device not found", "Device parameter error", "Device unit error", "Cannot open device", "Device call aborted", "Generic error", "Cancelled by user", "Object ID too low", "Object ID too high", "Object not in heap", "Unknown heap", "Unknown object (invalid DefProc)", "Unknown object (DefProc not in table)", "Message out of range", "Invalid (null) method", "Unknown message", "Manager call not supported", "Bad address", "Network operation in progress", "Network operation timed out", "Connection is busy", "Network attribute not supported", "Network error", "Address in use", "System out of memory", "Connection aborted", "Connection refused", "Not connected", "Already connected", "Connection closed", "Initialization error (interapplication manager)", "Bad occurrence", "Wait on unbound occurrence handler", "Occurrence queue overflow", "Datalog type conflict", "Unused", "Unrecognized type (interapplication manager)", "Memory corrupt", "Failed to make temporary DLL", "Old CIN version", "Drag socket not found", "Failed to load drop-object", "Failed to register OLE object", "Failed to release OLE object", "Format specifier type mismatch", "Unknown format specifier", "Too few format specifiers", "Too many format specifiers", "Scan failed", "Newer CIN version", "Error converting to variant", "Runtime menu error", "Password tampered", "Variant attribute not found", "Incompatible variant data type", "Event data is not available", "Event Store is not present", "Occurrence is not found", "Event Queue is not created", "Event info is not available", "Refnum passed is NULL", "Error retrieving Class GUID", "Error retrieving CoClass GUID", "Error retrieving TypeLib GUID.", "Bad built application magic bytes.", "Specific driver is different from the specific driver associated with the Logical Name.", "There is no session opened to the class driver.", "Max Error", "MAX - Error with config objects", "MAX - Error loading configuration", "MAX - Group not supported"]
        # "Current State"
        # "Do not delete, rename, or modify this frame.\n(this is used to capture unhandled states and typos)"
        # "Handle mistyped state name (developer tool)"
        n43 = Format Into String(format string="Software Exception: Unhandled State \"%s\"." ("message"), error in=w101, w96) -> (resulting string=w104:string, error out=w103:errorcluster)  [unwired: 1 in]
        n44 = call <vilib>:"Error Cluster From Error Code.vi"("show call chain? (False)"=TRUE, "error in (no error)"=w103, "error message (\"\")"=w104, "error code (0)"=w105) -> ("error out"=w102:errorcluster)  [unwired: 5 in]
        n45 = call <vilib>:"Add State(s) to Queue__JKI_lib_State_Machine.vi"("State(s) in (\"\")"=w100) -> ("States Out"=w99:string)  [unwired: 14 in]
      }
      frame "Initialize Core Data" {
        # "Do not delete, rename, or modify this frame.\n(this is used to determine panel behavior on exit)"
        # "originally closed?"
        # "exe?"
        # "If panel starts closed or is an EXE, then close it when we exit"
        n46 = property class="VI"() -> ("Front Panel.Open"=w114:bool)  [unwired: 2 in, 2 out]
        n47 = property class="App"() -> ("App.Kind"=w113:T1)  [unwired: 2 in, 2 out]
        n48 = control-ref of="Current VI Reference"() -> (w107:refnum<vi>)
        n49 = Not(x=w114) -> (.not. x?=w111:bool)
        n50 = Equal?(x=w113, y=T1."Run Time System" ("Application:Kind")) -> (x = y?=w110:bool)
        n51 = Or(x=w111, y=w110) -> (x .or. y?=w108:bool)
        n52 = Bundle By Name(cluster=w109, "Core.Current VI Reference"=w107, "Core.Close Panel on Exit?"=w108) -> (w116:T3)
        n53 = call <vilib>:"Add State(s) to Queue__JKI_lib_State_Machine.vi"("State(s) in (\"\")"=w118) -> ("States Out"=w117:string)  [unwired: 14 in]
      }
      frame "Error Handler" {
        # "Unhandled Error -- Display it"
        # "Handle any errors here.\nYou can also output any states to clean-up after errors occur"
        # "Clear error"
        n54 = call <vilib>:"General Error Handler.vi"("error in (no error)"=w120) -> ()  [unwired: 10 in, 5 out]
        n55 = call <vilib>:"Add State(s) to Queue__JKI_lib_State_Machine.vi"("State(s) in Front (\"\")"="/* Post Error States", "State(s) in (\"\")"=w124) -> ("States Out"=w123:string)  [unwired: 13 in]
      }
      frame "Exit" {
        # "Do not put any code in this frame.\n(No errors that occur here will be handled.)"
        n56 = call <vilib>:"Add State(s) to Queue__JKI_lib_State_Machine.vi"("State(s) in (\"\")"=w129) -> ("States Out"=w128:string)  [unwired: 14 in]
      }
      frame "---------- Data ----------" {
        # "Do not put any code in this frame.\n(It is a separator no-op. You can make a copy of this frame to create a new Data frame)"
        n57 = call <vilib>:"Add State(s) to Queue__JKI_lib_State_Machine.vi"("State(s) in (\"\")"=w133) -> ("States Out"=w132:string)  [unwired: 14 in]
      }
      frame "Data: Initialize" {
        w134 = FALSE  # 是否进行预警
        w135 = FALSE  # 是否进行预判
        w136 = T4 {"绘图坐标X"="", "绘图坐标Y"="", "实际坐标"=["415", "97342.968", "85485.997"]}  # 坐标关系
        w137 = ""  # Area_name
        w138 = 0  # 插值方式
        w139 = ""  # SampleTime
        w140 = string[][] [["101", "39", "0", "10"], ["102", "37", "0", "10"], ["103", "40", "2", "10"], ["104", "38", "2", "10"], ["105", "36", "2", "10"], ["106", "41", "4", "10"], ["107", "39", "4", "10"], ["108", "37", "4", "10"], ["109", "35", "4", "10"], ["110", "40", "6", "10"], ["111", "36", "6", "10"], ["112", "41", "8", "10"], ["113", "39", "8", "10"], ["114", "37", "8", "10"], ["115", "35", "8", "10"], ["116", "40", "10", "10"], ["117", "38", "10", "10"], ["118", "36", "10", "10"], ["119", "34", "10", "10"], ["120", "39", "12", "10"], ["121", "37", "12", "10"], ["122", "40", "14", "10"], ["123", "38", "14", "10"], ["124", "36", "14", "10"], ["125", "41", "16", "10"], ["126", "39", "16", "10"], ["127", "37", "16", "10"], ["128", "35", "16", "10"], ["129", "40", "18", "10"], ["130", "36", "17.75", "10"], ["131", "70", "0", "10"], ["132", "60", "0", "10"], ["133", "50", "0", "10"], ["134", "40", "8", "10"], ["135", "32", "8", "10"], ["136", "40", "0", "10"], ["137", "32", "0", "10"], ["138", "40", "8", "10"], ["139", "32", "8", "10"], ["140", "40", "0", "10"], ["141", "70", "0", "10"], ["142", "60", "0", "10"], ["201", "33", "0", "10"], ["202", "31", "0", "10"], ["203", "34", "2", "10"], ["204", "32", "2", "10"], ["205", "30", "2", "10"], ["206", "28", "2", "10"], ["207", "33", "4", "10"], ["208", "31", "4", "10"], ["209", "29", "4", "10"], ["210", "27", "4", "10"], ["211", "34", "6", "10"], ["212", "30", "6", "10"], ["213", "28", "6", "10"], ["214", "33", "8", "10"], ["215", "31", "8", "10"], ["216", "29", "8", "10"], ["217", "27", "8", "10"], ["218", "32", "10", "10"], ["219", "30", "10", "10"], ["220", "28", "10", "10"], ["221", "33", "12", "10"], ["222", "31", "12", "10"], ["223", "34", "14", "10"], ["224", "32", "14", "10"], ["225", "30", "14", "10"], ["226", "28", "14", "10"], ["227", "33", "16", "10"], ["228", "31", "16", "10"], ["229", "29", "16", "10"], ["230", "34", "17.5", "10"], ["231", "30", "17", "10"], ["232", "28", "17", "10"], ["233", "40", "0", "10"], ["234", "30", "0", "10"], ["235", "24", "8", "10"], ["236", "16", "8", "10"], ["237", "24", "0", "10"], ["238", "16", "0", "10"], ["239", "24", "8", "10"], ["240", "32", "0", "10"], ["241", "24", "0", "10"], ["242", "16", "0", "10"], ["243", "50", "0", "10"], ["244", "40", "0", "10"], ["245", "30", "0", "10"], ["301", "23", "27", "10"], ["302", "24", "25", "10"], ["303", "25", "21", "10"], ["304", "26", "19", "10"], ["305", "27", "26", "10"], ["306", "28", "24", "10"], ["307", "29", "22", "10"], ["308", "30", "20", "10"], ["309", "31", "18", "10"], ["310", "32", "25", "0"], ["311", "33", "23", "0"], ["312", "34", "21", "0"], ["313", "35", "19", "0"], ["314", "36", "17", "0"], ["315", "37", "24", "0"], ["316", "38", "22", "0"], ["317", "39", "18", "0"], ["318", "40", "25", "0"], ["319", "41", "23", "0"], ["320", "42", "21", "0"], ["321", "43", "19", "0"], ["322", "44", "26", "0"], ["323", "45", "24", "0"], ["324", "46", "22", "0"], ["325", "47", "20", "0"], ["326", "48", "18", "0"], ["327", "49", "27", "0"], ["328", "50", "25", "0"], ["329", "51", "21", "0"], ["330", "52", "19", "0"], ["331", "53", "26", "0"], ["332", "54", "24", "0"], ["333", "55", "22", "0"], ["334", "56", "20", "0"], ["335", "57", "27", "0"], ["336", "58", "25", "0"], ["337", "59", "23", "0"], ["338", "60", "21", "0"], ["339", "61", "19", "0"], ["340", "24", "17", "0"], ["341", "22", "17", "0"], ["342", "18", "17.5", "0"], ["401", "15", "0", "0"], ["402", "13", "0", "0"], ["403", "16", "2", "0"], ["404", "14", "2", "0"], ["405", "12", "2", "0"], ["406", "15", "4", "0"], ["407", "13", "4", "0"], ["408", "11", "4", "0"], ["409", "16", "6", "0"], ["410", "12", "6", "0"], ["411", "47", "8", "0"], ["412", "15", "8", "0"], ["413", "13", "8", "0"], ["414", "11", "8", "0"], ["415", "16", "10", "0"], ["416", "14", "10", "0"], ["417", "12", "10", "0"], ["418", "10", "10", "0"], ["419", "15", "12", "0"], ["420", "13", "12", "0"], ["421", "18", "14", "0"], ["422", "16", "14", "0"], ["423", "14", "14", "0"], ["424", "12", "14", "0"], ["425", "17", "16", "0"], ["426", "15", "16", "0"], ["427", "13", "16", "0"], ["428", "16", "17.5", "0"], ["429", "12", "18", "0"], ["430", "10", "18", "0"], ["431", "30", "0", "0"], ["432", "20", "0", "0"], ["433", "0", "0", "0"], ["434", "8", "0", "0"], ["435", "0", "0", "0"], ["436", "16", "8", "0"], ["437", "8", "8", "0"], ["438", "0", "8", "0"], ["439", "20", "0", "0"], ["440", "10", "0", "0"], ["441", "0", "0", "0"], ["501", "10", "2", "0"], ["502", "8", "2", "0"], ["503", "6", "2", "0"], ["504", "4", "2", "0"], ["505", "2", "2", "0"], ["506", "0", "2", "0"], ["507", "9", "4", "0"], ["508", "7", "4", "0"], ["509", "5", "4", "0"], ["510", "3", "4", "0"], ["511", "1", "4", "0"], ["512", "10", "6", "0"], ["513", "6", "6", "0"], ["514", "4", "6", "0"], ["515", "2", "6", "0"], ["516", "0", "6", "0"], ["517", "9", "8", "0"], ["518", "7", "8", "0"], ["519", "5", "8", "0"], ["520", "3", "8", "0"], ["521", "1", "8", "0"], ["522", "8", "10", "0"], ["523", "6", "10", "0"], ["524", "4", "10", "0"], ["525", "2", "10", "0"], ["526", "0", "10", "0"], ["527", "9", "12", "0"], ["528", "7", "12", "0"], ["529", "3", "12", "0"], ["530", "1", "12", "0"], ["531", "0", "18", "0"], ["532", "10", "14", "0"], ["533", "8", "14", "0"], ["534", "6", "14", "0"], ["535", "4", "14", "0"], ["536", "2", "14", "0"], ["537", "0", "14", "0"]]  # 采样数据
        w141 = FALSE  # 是否存在记录
        w142 = cluster{"X":dbl[], "Y":dbl[], "Z":dbl[]} {"X"=[], "Y"=[], "Z"=[]}  # 3DData
        w143 = T5 {"Current VI Reference"=refnum, "Close Panel on Exit?"=FALSE}  # Core
        w145 = TRUE  # Your Boolean data
        w144 = ""  # Your string data
        # "do not delete - used by framework"
        # "Data names and types of shift register data are defined by this bundle."
        # "Initialize the shift-register data, here.\n(data names are defined by what you wire into the bundle function)"
        n58 = Bundle("Core"=w143, "Your Boolean data"=w145, "Your string data"=w144, "3DData"=w142, "是否存在记录"=w141, "采样数据"=w140, "SampleTime"=w139, "插值方式"=w138, "Area_name"=w137, "坐标关系"=w136, "是否进行预判"=w135, "是否进行预警"=w134) -> (w147:T3)  [unwired: 1 in]
        n59 = call <vilib>:"Add State(s) to Queue__JKI_lib_State_Machine.vi"("State(s) in (\"\")"=w149) -> ("States Out"=w148:string)  [unwired: 14 in]
      }
      frame "Data: Cleanup" {
        # "Cleanup any data and references, here.\n(this is called automatically, by the Macro: Exit)"
        n60 = Unbundle By Name(w150) -> ("Core.Current VI Reference"=w153:refnum<vi>)
        n61 = Close Reference(reference=w153, error in (no error)=w152) -> (error out=w151:errorcluster)
        n62 = call <vilib>:"Add State(s) to Queue__JKI_lib_State_Machine.vi"("State(s) in (\"\")"=w155) -> ("States Out"=w154:string)  [unwired: 14 in]
      }
      frame "---------- UI ----------" {
        # "Do not put any code in this frame.\n(It is a separator no-op. You can make a copy of this frame to create a new UI frame)"
        n63 = call <vilib>:"Add State(s) to Queue__JKI_lib_State_Machine.vi"("State(s) in (\"\")"=w159) -> ("States Out"=w158:string)  [unwired: 14 in]
      }
      frame "UI: Initialize" {
        w160 = ""
        (unwired) "3D:Drawing3DSurfaceGraph"
        # "Initialize the User Interface, here.\n(this is called automatically, by the Macro: Init)"
        n64 = local write "导出数据位置"(path "" ("导出数据位置")) -> ()
        n65 = local write "预判点"(w160) -> ()
        n66 = local write "渗漏点"(w160) -> ()
        n67 = call <vilib>:"Add State(s) to Queue__JKI_lib_State_Machine.vi"("State(s) in (\"\")"=w165) -> ("States Out"=w164:string)  [unwired: 14 in]
      }
      frame "UI: Cursor Set" {
        # "Argument"
        # "Set and Unset Cursor Busy.\n(Usage: \"UI: Cursor Set >> Busy|Idle\")"
        n68 = case shown="\"Idle\", 默认" w166 {
          tunnel: w168 -> [w173 w175]
          tunnel: [w172 w174] -> w167
          frame "Idle", Default {
            n69 = call <vilib>:"Unset Busy.vi"("error in (no error)"=w173) -> ("error out"=w172:errorcluster)  [unwired: 10 in]
          }
          frame "Busy" {
            n70 = call <vilib>:"Set Busy.vi"("error in (no error)"=w175) -> ("error out"=w174:errorcluster)  [unwired: 9 in, 1 out]
          }
        }
        n71 = call <vilib>:"Add State(s) to Queue__JKI_lib_State_Machine.vi"("State(s) in (\"\")"=w171) -> ("States Out"=w170:string)  [unwired: 14 in]
      }
      frame "UI: Front Panel State" {
        # "Argument"
        # "Set Front Panel Open or Closed\n(Usage: \"UI: Front Panel State >> Open|Close\")"
        n72 = Unbundle By Name(w178) -> ("Core.Current VI Reference"=w177:refnum<vi>)
        n73 = case shown="\"Open\", 默认" w176 {
          tunnel: w180 -> [w186 w199]
          tunnel: [w188 w200] -> w179
          tunnel: w177 -> [w187 w197]
          frame "Open", Default {
            n74 = property class="VI"(reference=w187, error in=w186) -> (reference out=w184:refnum<vi>, error out=w185:errorcluster, "Front Panel.Open"=w183:bool)
            n75 = case shown="假" w183 {
              tunnel: [w191 w194] -> w188
              tunnel: w185 -> [w190 w194]
              tunnel: w184 -> [w189 _]
              frame False {
                n76 = invoke class="VI" method="FP.Open"(reference=w189, error in=w190, "Activate"=TRUE, "State"=T2."Standard") -> (error out=w191:errorcluster)  [unwired: 1 in, 4 out]
              }
              frame True {
              }
            }
          }
          frame "Close" {
            n77 = property class="VI"(reference=w197, error in=w199) -> (reference out=w196:refnum<vi>, error out=w198:errorcluster, "Front Panel.Open"=w195:bool)
            n78 = case shown="真" w195 {
              tunnel: [w201 w204] -> w200
              tunnel: w198 -> [w201 w203]
              tunnel: w196 -> [_ w202]
              frame False {
              }
              frame True {
                n79 = invoke class="VI" method="FP.Close"(reference=w202, error in=w203) -> (error out=w204:errorcluster)  [unwired: 1 in, 2 out]
              }
            }
          }
        }
        n80 = call <vilib>:"Add State(s) to Queue__JKI_lib_State_Machine.vi"("State(s) in (\"\")"=w182) -> ("States Out"=w181:string)  [unwired: 14 in]
      }
      frame "---------- Macro ----------" {
        # "Do not put any code in this frame.\n(It is a separator no-op. You can make a copy of this frame to create a new Macro frame)"
        n81 = call <vilib>:"Add State(s) to Queue__JKI_lib_State_Machine.vi"("State(s) in (\"\")"=w208) -> ("States Out"=w207:string)  [unwired: 14 in]
      }
      frame "Macro: Initialize" {
        w212 = "Data: Initialize\nInitialize Core Data\nUI: Initialize\nUI: Front Panel State >> Open\n3D:Get3DData\n3D:Drawing3DMeshGraph\n3D:Drawing3DContourGraph\n3D:Drawing3DSurfaceGraph"  # Data: Initialize Initialize Core Data UI: Initialize UI: Front Panel State >> Open 3D:Get3DData 3D:Drawing3DMeshGraph 3D:Drawing3DContourGraph 3D:Drawing3DSurfaceGraph
        # "Initialization Macro\n(This is called once, when the VI starts)"
        n82 = Bundle By Name(cluster=w210, "是否进行预判"=FALSE) -> (w209:T3)
        n83 = call <vilib>:"Add State(s) to Queue__JKI_lib_State_Machine.vi"("State(s) in Front (\"\")"=w212, "State(s) in (\"\")"=w215) -> ("States Out"=w214:string)  [unwired: 13 in]
      }
      frame "Macro: Exit" {
        (unwired) FALSE
        # "Exit Macro\n(This is called once, when the VI exits)"
        n84 = Unbundle By Name(w225) -> ("Core.Close Panel on Exit?"=w224:bool)
        n85 = Bundle(u32 65295, u32 65295) -> (w217:cluster{u32, u32})  [unwired: 1 in]
        n86 = Build Array(w217) -> ()  [unwired: 1 out]
        n87 = Select(t="UI: Front Panel State >> Close", s=w224, f="") -> (s? t:f=w221:string)
        n88 = call <vilib>:"Add State(s) to Queue__JKI_lib_State_Machine.vi"("State(s) in (\"\")"=w221, "State(s) at Back (\"\")"="Data: Cleanup\nExit") -> ("States Out"=w219:string)  [unwired: 13 in]
        n89 = call <vilib>:"Add State(s) to Queue__JKI_lib_State_Machine.vi"("State(s) in Front (\"\")"=w219, "State(s) in (\"\")"=w228) -> ("States Out"=w227:string)  [unwired: 13 in]
      }
      frame "---------- New Category ----------" {
        # "Template Separator\n(You can make a copy of, or modify, this frame)"
        n90 = call <vilib>:"Add State(s) to Queue__JKI_lib_State_Machine.vi"("State(s) in (\"\")"=w232) -> ("States Out"=w231:string)  [unwired: 14 in]
      }
      frame "New Category: 1" {
        # "Your code here.\n(You can make a copy of, or modify, this frame)"
        n91 = call <vilib>:"Add State(s) to Queue__JKI_lib_State_Machine.vi"("State(s) in (\"\")"=w236) -> ("States Out"=w235:string)  [unwired: 14 in]
      }
      frame "New Category: 2" {
        # "Your code here.\n(You can make a copy of, or modify, this frame)"
        n92 = call <vilib>:"Add State(s) to Queue__JKI_lib_State_Machine.vi"("State(s) in (\"\")"=w240) -> ("States Out"=w239:string)  [unwired: 14 in]
      }
      frame "----------fenxishuju----------" {
        # "Your code here.\n(You can make a copy of, or modify, this frame)"
        n93 = call <vilib>:"Add State(s) to Queue__JKI_lib_State_Machine.vi"("State(s) in (\"\")"=w244) -> ("States Out"=w243:string)  [unwired: 14 in]
      }
      frame "fenxishuju:预警" {
        # "删除最小值"
        # "删除最大值"
        # "Your code here.\n(You can make a copy of, or modify, this frame)"
        n94 = Unbundle By Name(w256) -> ("3DData.Z"=w253:dbl[])  [unwired: 1 out]
        n95 = Array Max & Min(array=w253) -> (max value=w247:dbl, max index (indices)=w254:i32, min index (indices)=w252:i32)  [unwired: 1 out]
        n96 = Delete From Array(array=w253, index=w254) -> (array with subset deleted=w251:dbl[])  [unwired: 1 in, 1 out]
        n97 = Delete From Array(array=w251, index=w252) -> (array with subset deleted=w249:dbl[])  [unwired: 1 in, 1 out]
        n98 = Array Size(array=w249) -> (size(s)=w248:i32)
        n99 = Add Array Elements(numeric array=w249) -> (sum=w250:dbl)
        n100 = Divide(x=w250, y=w248) -> (x/y=w246:dbl)
        n101 = case shown="真" TRUE {
          tunnel: w256 -> [w263 w268]
          tunnel: [w262 w266] -> w255
          tunnel: w247 -> [_ w265]
          tunnel: w246 -> [_ w264]
          frame False {
            n102 = Bundle By Name(cluster=w263, "是否进行预警"=FALSE) -> (w262:T3)
            n103 = One Button Dialog(message="没有预判和渗漏分析，无法预警") -> ()  [unwired: 1 in, 1 out]
          }
          frame True {
            n104 = disable-structure shown="禁用" {
              disable-tunnel: w265 -> [w273 _]
              disable-tunnel: w264 -> [w272 _]
              frame Disabled {
                n105 = Quotient & Remainder(x=w273, y=w272) -> (floor(x/y)=w271:dbl)  [unwired: 1 out]
                n106 = Round To Nearest(number=w271) -> (nearest integer value=w270:dbl)
                n107 = case shown="8.." w270 {
                  tunnel: [enum16{"红", "黄", "橙", "绿"}."绿" ("预警颜色") enum16{"红", "黄", "橙", "绿"}."绿" ("预警颜色") enum16{"红", "黄", "橙", "绿"}."绿" ("预警颜色") enum16{"红", "黄", "橙", "绿"}."绿" ("预警颜色") enum16{"红", "黄", "橙", "绿"}."橙" ("预警颜色") enum16{"红", "黄", "橙", "绿"}."橙" ("预警颜色") enum16{"红", "黄", "橙", "绿"}."红" ("预警颜色") enum16{"红", "黄", "橙", "绿"}."红" ("预警颜色") enum16{"红", "黄", "橙", "绿"}."红" ("预警颜色")] -> w269
                  frame 0, Default {
                  }
                  frame 1 {
                  }
                  frame 2 {
                  }
                  frame 3 {
                  }
                  frame 4 {
                  }
                  frame 5 {
                  }
                  frame 6 {
                  }
                  frame 7 {
                  }
                  frame 8.. {
                  }
                }
                n108 = case shown="\"红\", 默认" w269 {
                  frame "红", Default {
                    n109 = Bundle(u32 13107200, u32 13107200) -> (w285:cluster{u32, u32})  [unwired: 1 in]
                    n110 = Build Array(w285) -> (w284:cluster{u32, u32}[])
                    n111 = property on="属性节点" class="Bool (严格)"("Colors [4]"=w284, "Blinking"=FALSE) -> ()  [unwired: 2 in, 2 out]
                  }
                  frame "橙" {
                    n112 = Bundle(u32 16742674, u32 15692544) -> (w290:cluster{u32, u32})  [unwired: 1 in]
                    n113 = Build Array(w290) -> (w289:cluster{u32, u32}[])
                    n114 = property on="属性节点" class="Bool (严格)"("Colors [4]"=w289, "Blinking"=FALSE) -> ()  [unwired: 2 in, 2 out]
                  }
                  frame "绿" {
                    (unwired) FALSE
                    n115 = Bundle(u32 65295, u32 65295) -> (w293:cluster{u32, u32})  [unwired: 1 in]
                    n116 = Build Array(w293) -> ()  [unwired: 1 out]
                  }
                }
              }
              frame Enabled {
              }
            }
            n117 = Bundle By Name(cluster=w268, "是否进行预警"=FALSE) -> (w266:T3)
          }
        }
        n118 = call <vilib>:"Add State(s) to Queue__JKI_lib_State_Machine.vi"("State(s) in (\"\")"=w259) -> ("States Out"=w258:string)  [unwired: 14 in]
      }
      frame "fenxishuju:quedingloudian" {
        # "Your code here.\n(You can make a copy of, or modify, this frame)"
        n119 = Unbundle By Name(w297) -> ("是否存在记录"=w299:bool, "采样数据"=w302:string[][], "插值方式"=w301:i32, "Area_name"=w300:string, "是否进行预判"=w298:bool)  [unwired: 3 out]
        n120 = case shown="真" w298 {
          tunnel: w302 -> [_ w323]
          tunnel: w301 -> [_ _]
          tunnel: w300 -> [_ w322]
          tunnel: w299 -> [_ w320]
          tunnel: [w306 w315] -> w296
          tunnel: w297 -> [w308 w314]
          frame False {
            n121 = One Button Dialog(message="没有预判，无法疑似点定位" ("消息")) -> ()  [unwired: 1 in, 1 out]
            n122 = Bundle By Name(cluster=w308, "是否进行预判"=FALSE) -> (w306:T3)
          }
          frame True {
            # "三维曲面图"
            n123 = disable-structure shown="禁用" {
              disable-tunnel: w322 -> [w616 _]
              frame Disabled {
                n124 = Format Into String(format string="select electrodes_gps_x,electrodes_gps_y from t_detection_electrodes  where area_name ='%s';", w616) -> (resulting string=w609:string)  [unwired: 2 in, 1 out]
                n125 = call "SelectData.vi"("SQL query"=w609) -> ("recordset data"=w619:variant[][])  [unwired: 7 in, 1 out]
                n126 = call "ReadDataFromDatabase.vi"("长度"=2, "index"=0, "recordset data"=w619) -> ("所有记录"=w612:string[][])  [unwired: 7 in, 1 out]
                n127 = Index Array(array=w612, index (col)=1) -> (element=w613:string[])  [unwired: 1 in]
                n128 = Index Array(array=w612, index (col)=0) -> (element=w611:string[])  [unwired: 1 in]
                n129 = Fract/Exp String To Number(string=w613) -> (number=→"数字 2":dbl[])  [unwired: 3 in, 1 out]
                n130 = Fract/Exp String To Number(string=w611) -> (number=→"数字":dbl[])  [unwired: 3 in, 1 out]
              }
              frame Enabled {
              }
            }
            n131 = call "IndexSampleData.vi"("SampleData"=w323) -> ("Y"=w317:dbl[], "X"=w319:dbl[], "Z"=w321:dbl[])  [unwired: 7 in, 1 out]
            n132 = Bundle By Name(cluster=w314, "是否进行预判"=FALSE, "是否进行预警"=TRUE) -> (w313:T3)
            n133 = Array Max & Min(array=w317) -> (max value=w316:dbl)  [unwired: 3 out]
            n134 = Array Max & Min(array=w319) -> (max value=w318:dbl)  [unwired: 3 out]
            n135 = case shown="真" w320 {
              tunnel: w317 -> [_ w336]
              tunnel: w319 -> [_ w335]
              tunnel: w321 -> [_ w334]
              tunnel: w318 -> [_ w329]
              tunnel: w316 -> [_ w328]
              tunnel: [w324 w326] -> w315
              tunnel: w313 -> [w324 w326]
              tunnel: 2 -> [_ w325]
              frame False {
              }
              frame True {
                n136 = mathscript code="n=4;\n%x=str2double(a)\n%y=str2double(b)\nnStepx = (Xmax+1)*n;\nnStepy = (Ymax+1)*n\n%nStepx = 400;\n%nStepy = 400;\nxi=linspace(min(a),max(a),nStepx);\nyi=linspace(min(b),max(b),nStepy);\n[Xi,Yi]=meshgrid(xi,yi);\nif czfs==0\n        Zi=griddata(a,b,c,Xi,Yi,'linear')\nelse if  czfs==1\n           Zi=griddata(a,b,c,Xi,Yi,'cubic')\n       else if czfs==2\n              Zi=griddata(a,b,c,Xi,Yi,'nearest')\n              end\n        end\nend"("a"=w335, "b"=w336, "c"=w334, "czfs"=w325, "Xmax"=w329, "Ymax"=w328) -> ("Zi"=w332:dbl[][], "n"=w331:i32)  [unwired: 1 in, 1 out]
                n137 = control-ref of="渗漏点"() -> (w333:refnum<vi>)
                n138 = Unbundle By Name(w326) -> ("坐标关系"=w327:T4)
                n139 = call "FindLeakPeak.vi"("坐标关系"=w327, "n 等分倍数"=w331, "Zi"=w332, "渗漏点"=w333) -> ("最大索引"=→"最大索引":u32[])  [unwired: 4 in, 3 out]
              }
            }
          }
        }
        n140 = call <vilib>:"Add State(s) to Queue__JKI_lib_State_Machine.vi"("State(s) in (\"\")"=w305) -> ("States Out"=w304:string)  [unwired: 14 in]
      }
      frame "fenxishuju:yupan" {
        # "select detection_electrodes_name,electrodes_gps_x,electrodes_gps_y from t_detection_electrodes where electrodes_map_x='%s',electrodes_map_y='%s';"
        # "三维曲面图"
        # "Your code here.\n(You can make a copy of, or modify, this frame)"
        n141 = control-ref of="预判点"() -> (w620:refnum<vi>)
        n142 = property class="Str"(reference=w620, "Text.TextColor"=u32 13107200) -> ()  [unwired: 1 in, 2 out]
        n143 = Unbundle By Name(w624) -> ("采样数据"=w639:string[][])  [unwired: 5 out]
        n144 = control-ref of="绘图坐标X"() -> (w637:refnum<vi>)
        n145 = control-ref of="绘图坐标Y"() -> (w636:refnum<vi>)
        n146 = control-ref of="Zmax"() -> (w638:refnum<vi>)
        n147 = call "IndexSampleData.vi"("SampleData"=w639) -> ("Y"=w635:dbl[], "X"=w634:dbl[], "Z"=w633:dbl[])  [unwired: 7 in, 1 out]
        n148 = call "FindLeakMapCoordinate.vi"("Y"=w635, "Z"=w633, "reference 4"=w638, "X"=w634, "reference 3"=w637, "reference输入"=w636, "String输入"=w620) -> ("X"=w626:string, "Y"=w625:string)  [unwired: 3 in]
        n149 = Format Into String(format string="select detection_electrodes_name,electrodes_gps_x,electrodes_gps_y from t_detection_electrodes where electrodes_map_x='%s' and electrodes_map_y='%s';", w626, w625) -> (resulting string=w631:string)  [unwired: 2 in, 1 out]
        n150 = call "SelectData.vi"("SQL query"=w631) -> ("recordset data"=w630:variant[][])  [unwired: 7 in, 1 out]
        n151 = call "ReadDataFromDatabase.vi"("长度"=3, "index"=0, "recordset data"=w630) -> ("一行记录"=w627:string[])  [unwired: 7 in, 1 out]
        n152 = Bundle By Name(cluster=w624, "坐标关系.绘图坐标X"=w626, "坐标关系.绘图坐标Y"=w625, "坐标关系.实际坐标"=w627, "是否进行预判"=TRUE) -> (w623:T3)
        n153 = call <vilib>:"Add State(s) to Queue__JKI_lib_State_Machine.vi"("State(s) in (\"\")"=w642) -> ("States Out"=w641:string)  [unwired: 14 in]
      }
      frame "--------Chazhi--------" {
        # "Your code here.\n(You can make a copy of, or modify, this frame)"
        n154 = call <vilib>:"Add State(s) to Queue__JKI_lib_State_Machine.vi"("State(s) in (\"\")"=w646) -> ("States Out"=w645:string)  [unwired: 14 in]
      }
      frame "Chazhi:GetChazhifangshi" {
        # "Your code here.\n(You can make a copy of, or modify, this frame)"
        n155 = Unbundle By Name(w648) -> ("插值方式"=w649:i32)
        n156 = Bundle By Name(cluster=w648, "插值方式"=w649) -> (w647:T3)
        n157 = call <vilib>:"Add State(s) to Queue__JKI_lib_State_Machine.vi"("State(s) in (\"\")"=w652) -> ("States Out"=w651:string)  [unwired: 14 in]
      }
      frame "----------Data--------" {
        # "Your code here.\n(You can make a copy of, or modify, this frame)"
        n158 = call <vilib>:"Add State(s) to Queue__JKI_lib_State_Machine.vi"("State(s) in (\"\")"=w656) -> ("States Out"=w655:string)  [unwired: 14 in]
      }
      frame "Data:ExportDataToCVS" {
        (unwired) path "C:/Users/craes/Desktop/小城故事/shuj.csv" ("file path (dialog if empty)")
        # "Your code here.\n(You can make a copy of, or modify, this frame)"
        n159 = flat-sequence {
          tunnel: w659 -> [w666]
          tunnel: [w666] -> w658
          tunnel: [w663] -> w657
          tunnel: w658 -> [w668]
          tunnel: w657 -> [w667]
          frame #0 {
            n160 = local write "选项卡控件"(3) -> ()
            n161 = Two Button Dialog(message="是否导出采样数据？" ("消息")) -> (T button?=w663:bool)  [unwired: 2 in]
          }
          frame #1 {
            n162 = case shown="真" w667 {
              tunnel: w668 -> [_ w693]
              frame False {
              }
              frame True {
                n163 = Current VI's Path() -> (path=w687:path)
                n164 = Strip Path(path=w687) -> (stripped path=w686:path)  [unwired: 1 out]
                n165 = Unbundle By Name(w693) -> ("采样数据"=w691:string[][], "SampleTime"=w676:string)  [unwired: 1 out]
                n166 = Strip Path(path=w686) -> (stripped path=w684:path)  [unwired: 1 out]
                n167 = Strip Path(path=w684) -> (stripped path=w683:path)  [unwired: 1 out]
                n168 = Path To String(path=w683) -> (string=w682:string)
                n169 = property on="采样数据" class="MCListbox (严格)"("ItemNames"=w691) -> ()  [unwired: 2 in, 2 out]
                n170 = String Subset(string=w676, length (rest)=10 ("长度（剩余）")) -> (substring=w672:string)  [unwired: 1 in]
                n171 = String Subset(string=w676, offset (0)=11, length (rest)=5) -> (substring=w675:string)
                n172 = property on="采样数据" class="MCListbox (严格)"() -> ("ColHdrString"=w690:string[])  [unwired: 2 in, 2 out]
                n173 = call <vilib>:"Space Constant.vi"() -> ("String"=w669:string)
                n174 = Search and Replace String(input string=w675, search string=":" ("搜索字符串"), replace string="-" ("替换字符串(\"\")")) -> (result string=w670:string)  [unwired: 5 in, 3 out]
                n175 = Concatenate Strings(w682, "\\", w672, w669, w670, "数据.csv") -> (w680:string)
                n176 = Insert Into Array(array=w691, index (row)=0 ("索引 (行)"), new element=w690) -> (w688:string[][])  [unwired: 1 in]
                n177 = Build Path(name or relative path=w680) -> (appended path=w681:path)  [unwired: 1 in]
                "导出数据位置" <- w681
                n178 = call-poly <vilib>:"Write To Spreadsheet File.vi"("delimiter (\\t)"="," ("delimiter (\\t)"), "2D data"=w688, "file path (dialog if empty)"=w681) -> ()  [unwired: 5 in, 1 out]
              }
            }
          }
        }
        n179 = call <vilib>:"Add State(s) to Queue__JKI_lib_State_Machine.vi"("State(s) in (\"\")"=w662) -> ("States Out"=w661:string)  [unwired: 14 in]
      }
      frame "--------------3D-------------" {
        # "Your code here.\n(You can make a copy of, or modify, this frame)"
        n180 = call <vilib>:"Add State(s) to Queue__JKI_lib_State_Machine.vi"("State(s) in (\"\")"=w697) -> ("States Out"=w696:string)  [unwired: 14 in]
      }
      frame "3D:DrawingMju" {
        # "Your code here.\n(You can make a copy of, or modify, this frame)"
        n181 = Unbundle By Name(w701) -> ("3DData.X"=w700:dbl[], "3DData.Y"=w699:dbl[], "3DData.Z"=w698:dbl[])
        n182 = mathscript code="% x,y,value,坐标向量\nnStep = 100;\nnStepx = 100;\nnStepy = 100;\n% nSept 等分数\nA = 9.75859;\nB = 6.37052;\nC = 0.017;\nD = 3.6693;\nE = 3.288;\nF = 1.0;\n\n\n%产生等分矩阵\nX = linspace(min(x), max(x), nStepx);\nY = linspace(min(y), max(y), nStepy);\n[XX,YY] =  meshgrid(X,Y);\n%计算每个点到电极点距离\nDec1 = zeros(nStepx,nStepy);\nDec2 = zeros(nStepx,nStepy);\nDec3 = zeros(nStepx,nStepy);\nDec4 = zeros(nStepx,nStepy);\nDec5 = zeros(nStepx,nStepy);\nDec6 = zeros(nStepx,nStepy);\nDec7 = zeros(nStepx,nStepy);\nfor i=1:7\n    RR = sqrt((XX-x(i)).*(XX-x(i))+(YY-y(i)).*(YY-y(i)));\n    CV = F*(A+B*exp(-1*RR/C) + D*exp(-1*RR/E));\n    %Dec(:,:,i) = (CV - abs(value(i)) ).*(CV - abs(value(i)) );\n  if i==1\n     Dec1(:,:)=(CV - abs(value(i)) ).*(CV - abs(value(i)) );\n  end\n  if i==2\n     Dec2(:,:)=(CV - abs(value(i)) ).*(CV - abs(value(i)) );\n  end\n  if i==3\n     Dec3(:,:)=(CV - abs(value(i)) ).*(CV - abs(value(i)) );\n  end\n  if i==4\n     Dec4(:,:)=(CV - abs(value(i)) ).*(CV - abs(value(i)) );\n  end\n  if i==5\n     Dec5(:,:)=(CV - abs(value(i)) ).*(CV - abs(value(i)) );\n  end\n  if i==6\n     Dec6(:,:)=(CV - abs(value(i)) ).*(CV - abs(value(i)) );\n  end\n  if i==7\n     Dec7(:,:)=(CV - abs(value(i)) ).*(CV - abs(value(i)) );\n  end\nend\n%去掉电极点坐标\nfor i=1:7\n    for j=1:nStep\n       if X(j)==x(i)\n           for m=1:nStep\n               if Y(m)==y(i)\n                  %Dec(j,m,i) = NaN;\n                  if i==1\n                      Dec1(j,m)=NaN;\n                  end\n                  if i==2\n                      Dec2(j,m)=NaN;\n                  end\n                  if i==3\n                      Dec3(j,m)=NaN;\n                  end\n                  if i==4\n                      Dec4(j,m)=NaN;\n                  end\n                  if i==5\n                      Dec5(j,m)=NaN;\n                  end\n                  if i==6\n                      Dec6(j,m)=NaN;\n                  end\n                  if i==7\n                      Dec7(j,m)=NaN;\n                  end\n                  \n               end\n             end\n        end\n    end\nend    \n%DecSum = Dec(:,:,1) +Dec(:,:,2) +Dec(:,:,3) +Dec(:,:,4) +Dec(:,:,5) +Dec(:,:,6) +Dec(:,:,7);\nDecSum = Dec1(:,:) +Dec2(:,:) +Dec3(:,:) +Dec4(:,:) +Dec5(:,:) +Dec6(:,:) +Dec7(:,:);\n%取出最大点    maxX,maxY---最大点索引，maxXi,maxYi---最大点坐标\n[maxDecR,maxR] = max(DecSum);\n[maxDec,maxX] = min(maxDecR);\nmaxY = maxR(maxX);\nmaxXiYi = [X(maxX),Y(maxY)]"("x"=w700, "y"=w699, "value"=w698) -> ()  [unwired: 1 in, 2 out]
        n183 = call <vilib>:"Add State(s) to Queue__JKI_lib_State_Machine.vi"("State(s) in (\"\")"=w704) -> ("States Out"=w703:string)  [unwired: 14 in]
      }
      frame "3D:Qingchu3DGraph" {
        # "Your code here.\n(You can make a copy of, or modify, this frame)"
        n184 = call <vilib>:"Add State(s) to Queue__JKI_lib_State_Machine.vi"("State(s) in (\"\")"=w2135) -> ("States Out"=w2134:string)  [unwired: 14 in]
      }
      frame "3D:Get3DData" {
        n185 = Bundle By Name(cluster=w2145, "采样数据"="采样数据", "3DData"="3DData", "是否存在记录"="是否存在记录", "SampleTime"="采样时间", "Area_name"="Area_name") -> (w2144:T3)
        n186 = property on="采样数据" class="MCListbox (严格)"("ItemNames"="采样数据") -> ()  [unwired: 2 in, 2 out]
        n187 = Concatenate Strings("采样时间：", "采样时间", "\r", "采样区域：", "Area_name") -> (w2136:string)
        n188 = property on="当前采样分析信息" class="Str"("Text.Text"=w2136) -> ()  [unwired: 2 in, 2 out]
        n189 = call <vilib>:"Add State(s) to Queue__JKI_lib_State_Machine.vi"("State(s) in (\"\")"=w2149) -> ("States Out"=w2148:string)  [unwired: 14 in]
      }
      frame "3D:Drawing3DContourGraph" {
        # "Your code here.\n(You can make a copy of, or modify, this frame)"
        n190 = Unbundle By Name(w2157) -> ("3DData.X"=w2151:dbl[], "3DData.Y"=w2150:dbl[], "3DData.Z"=w2152:dbl[], "是否存在记录"=w2156:bool, "插值方式"=w2153:i32)
        n191 = Array Max & Min(array=w2150) -> (max value=w2154:dbl)  [unwired: 3 out]
        n192 = Array Max & Min(array=w2151) -> (max value=w2155:dbl)  [unwired: 3 out]
        n193 = case shown="真" w2156 {
          tunnel: w2151 -> [_ w2170]
          tunnel: w2150 -> [_ w2169]
          tunnel: w2152 -> [_ w2168]
          tunnel: w2155 -> [_ w2164]
          tunnel: w2154 -> [_ w2163]
          tunnel: w2153 -> [_ w2162]
          frame False {
          }
          frame True {
            n194 = mathscript code="n=4;\nnStepx = (Xmax+1)*n;\nnStepy = (Ymax+1)*n\nxi=linspace(min(a),max(a),nStepx);\nyi=linspace(min(b),max(b),nStepy);\n[Xi,Yi]=meshgrid(xi,yi);\nif czfs==0\n        Zi=griddata(a,b,c,Xi,Yi,'linear')\nelse if  czfs==1\n           Zi=griddata(a,b,c,Xi,Yi,'cubic')\n       else if czfs==2\n              Zi=griddata(a,b,c,Xi,Yi,'nearest')\n              end\n        end\nend"("a"=w2170, "b"=w2169, "c"=w2168, "Xmax"=w2164, "Ymax"=w2163, "czfs"=w2162) -> ("Xi"=w2166:dbl[][], "Yi"=w2165:dbl[][], "Zi"=w2161:dbl[][])  [unwired: 1 in, 1 out]
            n195 = call-poly <vilib>:"Plot Helper.vi"("z matrix"=w2161, "y matrix"=w2165, "x matrix"=w2166) -> ("3D Plot lvclass Array out"=→"3D等高线":refnum<class "3D Plot Datatype.lvclass">[])  [unwired: 3 in, 5 out]
          }
        }
        n196 = call <vilib>:"Add State(s) to Queue__JKI_lib_State_Machine.vi"("State(s) in (\"\")"=w2160) -> ("States Out"=w2159:string)  [unwired: 14 in]
      }
      frame "3D:Drawing3DSurfaceGraph" {
        # "三维曲面图"
        # "Your code here.\n(You can make a copy of, or modify, this frame)"
        n197 = Unbundle By Name(w2450) -> ("3DData.X"=w2445:dbl[], "3DData.Y"=w2444:dbl[], "3DData.Z"=w2443:dbl[], "是否存在记录"=w2449:bool, "插值方式"=w2448:i32)
        n198 = Array Max & Min(array=w2444) -> (max value=w2446:dbl)  [unwired: 3 out]
        n199 = Array Max & Min(array=w2445) -> (max value=w2447:dbl)  [unwired: 3 out]
        n200 = case shown="真" w2449 {
          tunnel: w2445 -> [_ w2463]
          tunnel: w2444 -> [_ w2462]
          tunnel: w2443 -> [_ w2461]
          tunnel: w2448 -> [_ w2457]
          tunnel: w2447 -> [_ w2455]
          tunnel: w2446 -> [_ w2454]
          frame False {
          }
          frame True {
            n201 = mathscript code="n=4;\nnStepx = (Xmax+1)*n;\nnStepy = (Ymax+1)*n\nxi=linspace(min(a),max(a),nStepx);\nyi=linspace(min(b),max(b),nStepy);\n[Xi,Yi]=meshgrid(xi,yi);\nif czfs==0\n        Zi=griddata(a,b,c,Xi,Yi,'linear')\nelse if  czfs==1\n           Zi=griddata(a,b,c,Xi,Yi,'cubic')\n       else if czfs==2\n              Zi=griddata(a,b,c,Xi,Yi,'nearest')\n              end\n        end\nend\n%mesh(Xi,Yi,Zi);\n%grid on\n%surfc(Xi,Yi,Zi);\nmaxValue=max(Zi)\n%maxX=max(a)\n%maxY=max(b)\n%maxVV=max(Zi)"("a"=w2463, "b"=w2462, "c"=w2461, "czfs"=w2457, "Xmax"=w2455, "Ymax"=w2454) -> ("Xi"=w2459:dbl[][], "Yi"=w2458:dbl[][], "Zi"=w2456:dbl[][])  [unwired: 1 in, 1 out]
            n202 = call-poly <vilib>:"Plot Helper.vi"("z matrix"=w2456, "y matrix"=w2458, "x matrix"=w2459) -> ("3D Plot lvclass Array out"=→"3D Surface":refnum<class "3D Plot Datatype.lvclass">[])  [unwired: 3 in, 5 out]
          }
        }
        n203 = call <vilib>:"Add State(s) to Queue__JKI_lib_State_Machine.vi"("State(s) in (\"\")"=w2453) -> ("States Out"=w2452:string)  [unwired: 14 in]
      }
      frame "------备份----" {
        # "三维曲面图"
        # "Your code here.\n(You can make a copy of, or modify, this frame)"
        n204 = Unbundle By Name(w2770) -> ("3DData.X"=w2765:dbl[], "3DData.Y"=w2764:dbl[], "3DData.Z"=w2763:dbl[], "是否存在记录"=w2769:bool, "插值方式"=w2768:i32)
        n205 = control-ref of="Zmax"() -> (w2762:refnum<vi>)
        n206 = control-ref of="X坐标"() -> (w2761:refnum<vi>)
        n207 = control-ref of="Y坐标"() -> (w2760:refnum<vi>)
        n208 = Array Max & Min(array=w2764) -> (max value=w2766:dbl)  [unwired: 3 out]
        n209 = Array Max & Min(array=w2765) -> (max value=w2767:dbl)  [unwired: 3 out]
        n210 = call "FindLeakMap.vi"("Y"=w2764, "Y坐标"=w2760, "Z"=w2763, "X坐标"=w2761, "X"=w2765, "Z最大值"=w2762) -> ()  [unwired: 6 in]
        n211 = case shown="真" w2769 {
          tunnel: w2765 -> [_ w2782]
          tunnel: w2764 -> [_ w2781]
          tunnel: w2763 -> [_ w2780]
          tunnel: w2768 -> [_ w2779]
          tunnel: w2767 -> [_ w2777]
          tunnel: w2766 -> [_ w2776]
          frame False {
          }
          frame True {
            n212 = mathscript code="n=4;\nnStepx = (Xmax+1)*n;\nnStepy = (Ymax+1)*n\nxi=linspace(min(a),max(a),nStepx);\nyi=linspace(min(b),max(b),nStepy);\n[Xi,Yi]=meshgrid(xi,yi);\nif czfs==0\n        Zi=griddata(a,b,c,Xi,Yi,'linear')\nelse if  czfs==1\n           Zi=griddata(a,b,c,Xi,Yi,'cubic')\n       else if czfs==2\n              Zi=griddata(a,b,c,Xi,Yi,'nearest')\n              end\n        end\nend\n%mesh(Xi,Yi,Zi);\n%grid on\n%surfc(Xi,Yi,Zi);\nmaxValue=max(Zi)\n%maxX=max(a)\n%maxY=max(b)\n%maxVV=max(Zi)"("a"=w2782, "b"=w2781, "c"=w2780, "czfs"=w2779, "Xmax"=w2777, "Ymax"=w2776) -> ("Zi"=w2778:dbl[][], "n"=w2774:i32)  [unwired: 1 in, 4 out]
            n213 = control-ref of="渗漏点"() -> (w2775:refnum<vi>)
            n214 = call "FindLeakPeak.vi"("n 等分倍数"=w2774, "Zi"=w2778, "渗漏点"=w2775) -> ()  [unwired: 5 in, 4 out]
          }
        }
        n215 = call <vilib>:"Add State(s) to Queue__JKI_lib_State_Machine.vi"("State(s) in (\"\")"=w2773) -> ("States Out"=w2772:string)  [unwired: 14 in]
      }
      frame "3D:Drawing3DMeshGraph" {
        # "三维曲面图"
        # "Your code here.\n(You can make a copy of, or modify, this frame)"
        n216 = Unbundle By Name(w3092) -> ("是否存在记录"=w3091:bool, "采样数据"=w3090:string[][], "插值方式"=w3089:i32)  [unwired: 3 out]
        n217 = call "IndexSampleData.vi"("SampleData"=w3090) -> ("Y"=w3085:dbl[], "X"=w3086:dbl[], "Z"=w3087:dbl[])  [unwired: 7 in, 1 out]
        n218 = Array Max & Min(array=w3086) -> (max value=w3088:dbl)  [unwired: 3 out]
        n219 = Array Max & Min(array=w3085) -> (max value=w3084:dbl)  [unwired: 3 out]
        n220 = case shown="真" w3091 {
          tunnel: w3085 -> [_ w3102]
          tunnel: w3086 -> [_ w3101]
          tunnel: w3087 -> [_ w3100]
          tunnel: w3089 -> [_ w3099]
          tunnel: w3088 -> [_ w3098]
          tunnel: w3084 -> [_ w3096]
          frame False {
          }
          frame True {
            n221 = mathscript code="n=4;\nnStepx = (Xmax+1)*n;\nnStepy = (Ymax+1)*n\nxi=linspace(min(a),max(a),nStepx);\nyi=linspace(min(b),max(b),nStepy);\n[Xi,Yi]=meshgrid(xi,yi);\nif czfs==0\n        Zi=griddata(a,b,c,Xi,Yi,'linear')\nelse if  czfs==1\n           Zi=griddata(a,b,c,Xi,Yi,'cubic')\n       else if czfs==2\n              Zi=griddata(a,b,c,Xi,Yi,'nearest')\n              end\n        end\nend"("a"=w3101, "b"=w3102, "c"=w3100, "Xmax"=w3098, "Ymax"=w3096, "czfs"=w3099) -> ("Xi"=w3104:dbl[][], "Yi"=w3103:dbl[][], "Zi"=w3097:dbl[][])  [unwired: 1 in, 2 out]
            n222 = call-poly <vilib>:"Plot Helper.vi"("z matrix"=w3097, "y matrix"=w3103, "x matrix"=w3104) -> ("3D Plot lvclass Array out"=→"3D Mesh":refnum<class "3D Plot Datatype.lvclass">[])  [unwired: 3 in, 5 out]
          }
        }
        n223 = call <vilib>:"Add State(s) to Queue__JKI_lib_State_Machine.vi"("State(s) in (\"\")"=w3095) -> ("States Out"=w3094:string)  [unwired: 14 in]
      }
      frame "3D:Drawing3DGraph" {
        # "Your code here.\n(You can make a copy of, or modify, this frame)"
        n224 = case shown="\"3DMesh\"" w3381 {
          tunnel: [w3386 w3387 w3388] -> w3380
          frame "3DSurface", Default {
            w3386 = enum32{"三维曲面图", "三维等高线图", "三维网格图"}."三维曲面图"  # 三维图
          }
          frame "3DContour" {
            w3387 = enum32{"三维曲面图", "三维等高线图", "三维网格图"}."三维等高线图"  # 三维图
          }
          frame "3DMesh" {
            w3388 = enum32{"三维曲面图", "三维等高线图", "三维网格图"}."三维网格图"  # 三维图
          }
        }
        n225 = property on="选项卡控件" class="TabCtl (严格)"("Value"=w3380) -> ()  [unwired: 2 in, 2 out]
        n226 = call <vilib>:"Add State(s) to Queue__JKI_lib_State_Machine.vi"("State(s) in (\"\")"=w3385) -> ("States Out"=w3384:string)  [unwired: 14 in]
      }
    }
  }
